vi "main.vi"() -> ()   [LabVIEW 2016]
doc: "Use this template to build a producer/consumer design pattern with events to produce queue items. Use this design pattern instead of the User Interface Event Handler pattern for user interfaces when you want to execute code asynchronously in response to an event without slowing the user interface responsiveness."
uses:
  Microscope_Settings.ctl
  Laser.ctl
  Time_microseconds.ctl
  Phase_Shift.ctl
  Mirror_Voltage.ctl
  Z_Offset.ctl
  Gain.ctl
  Tuneable_Lens_Numeric_Control.ctl
  Piezo_micrometres.ctl
  waveforms.ctl
  Piezo_micrometres_slider_control.ctl
  Mirror_Gain_Slider_Control.ctl
  Tunable_Lens_Slider_Control.ctl
  Desktop/SPIM Controller/functions/Arduino/Old/ArduinoIII Older/MasterArduinoctl.ctl
  Desktop/SPIM Controller/functions/Arduino/Old/ArduinoIII Older/ArduinoII.ctl
panel:
  in  "Experiment Runs":dbl=1.0
  out "error out":errorcluster
  in  "Experiment?":bool
  in  "t2":dbl
  in  "t1":dbl
  in  "COM port":i32
  in  "Mode":T1(ring)
  in  "Number of Repetitions":u16=1 min=1 step=1
  in  "Time Interval  Between Repeats (µS)":T2 step=2
  in  "StopMultiDScan":bool
  in  "StartMultiDScan":bool
  in  "Number of Z Slices":i16=1 min=1 step=1
  in  "Z Mirror Control":enum16{"manual", "automatic"}(ring)
  in  "Apply ex/det correction":enum16{"no", "yes"}(ring)
  out "Z Mirror Voltage":T3 min=-10.0 max=10.0
  out "Adjusted Scan Mirror Voltage":T3 min=-10.0 max=10.0
  in  "set@minZ":bool
  in  "set@maxZ":bool
  in  "@ min Z":T3 min=-10.0 max=10.0
  in  "@ max Z":T3 min=-10.0 max=10.0
  in  "PiezoEndMicrometres":T4 caption="End (µm)" min=0.0 max=100.0
  in  "PiezoStartMicrometres":T4 caption="Start (µm)" min=0.0 max=100.0
  in  "setPiezoEnd":bool
  in  "setPiezoStart":bool
  in  "Lens 2":T5 min=0.0 max=3.0 step=0.0001 scale=0.0..3.0
  in  "Lens 1":T5 min=0.0 max=3.0 step=0.0001 scale=0.0..3.0
  in  "saveMicroscopeSettings":bool
  in  "applyCurrentMicroscopeSettings":bool
  in  "deleteCurrentMicroscopeSettings":bool
  in  "loadMicroscopeSettings":bool
  in  "addMicroscopeSettings":bool
  in  "Z Mirror Gain":T6 min=-10.0 max=10.0 scale=-0.1..0.1
  in  "Mirror Offset":dbl(slide) min=-10.0 max=10.0 step=0.01 scale=0.0..1.8
  in  "Laser":T7
  in  "Piezo Position (µm)":T8 min=0.0 max=100.0 scale=0.0..100.0
  in  "Mirror Voltage":dbl(slide) min=-10.0 max=10.0 step=0.01 scale=-4.0..5.0
  in  "setPosition2":bool
  in  "setPosition1":bool
  in  "Z offset 2":T9
  in  "Z offset 1":T9
  in  "Scan Mirror 2":T3 min=-10.0 max=10.0
  in  "Scan Mirror 1":T3 min=-10.0 max=10.0
  in  "setScanMirrorMin":bool
  in  "setScanMirrorMax":bool
  in  "MinScanMirror":T3 caption="Min" min=-10.0 max=10.0
  in  "MaxScanMirror":T3 caption="Max" min=-10.0 max=10.0
  in  "Offset":T3 min=-10.0 max=10.0
  in  "Amplitude":T3 min=-10.0 max=10.0
  in  "Phase Shift (µS)":i32(slide) scale=-5000.0..1000.0
  in  "Sweep Interval (µS)":T2 step=2
  in  "Sweep Time (µS)":T2 step=20
  in  "Microscope Settings":T10[](array[typedef]) {"Number Z Slices" min=1 step=1; "Piezo End (µm)" min=0.0 max=100.0; "Piezo Start (µm)" min=0.0 max=100.0; "Beam @ max Z" min=-10.0 max=10.0; "Beam @ min Z" min=-10.0 max=10.0; "Tuneable Lens 2" min=0.0 max=3.0 step=0.0001; "Tuneable Lens 1" min=0.0 max=3.0 step=0.0001; "Scan Mirror Position 2" min=-10.0 max=10.0; "Scan Mirror Position 1" min=-10.0 max=10.0; "Scan Mirror Amplitude" min=-10.0 max=10.0; "Scan Mirror Min" min=-10.0 max=10.0; "Scan Mirror Max" min=-10.0 max=10.0; "Sweep Interval (µS)" step=2; "Sweep Time (µS)" step=2}
  in  "Sample Rate (kHz)":i32
  in  "StopSinglePlaneScan":bool
  in  "StartSinglePlaneScan":bool
  in  "exit":bool
  # "Piezo Settings"
  # "Scan Mirror Settings"
  # "Z Mirror Local Settings"
  # "Single Plane Scan"
  # "Multidimensional Scan"
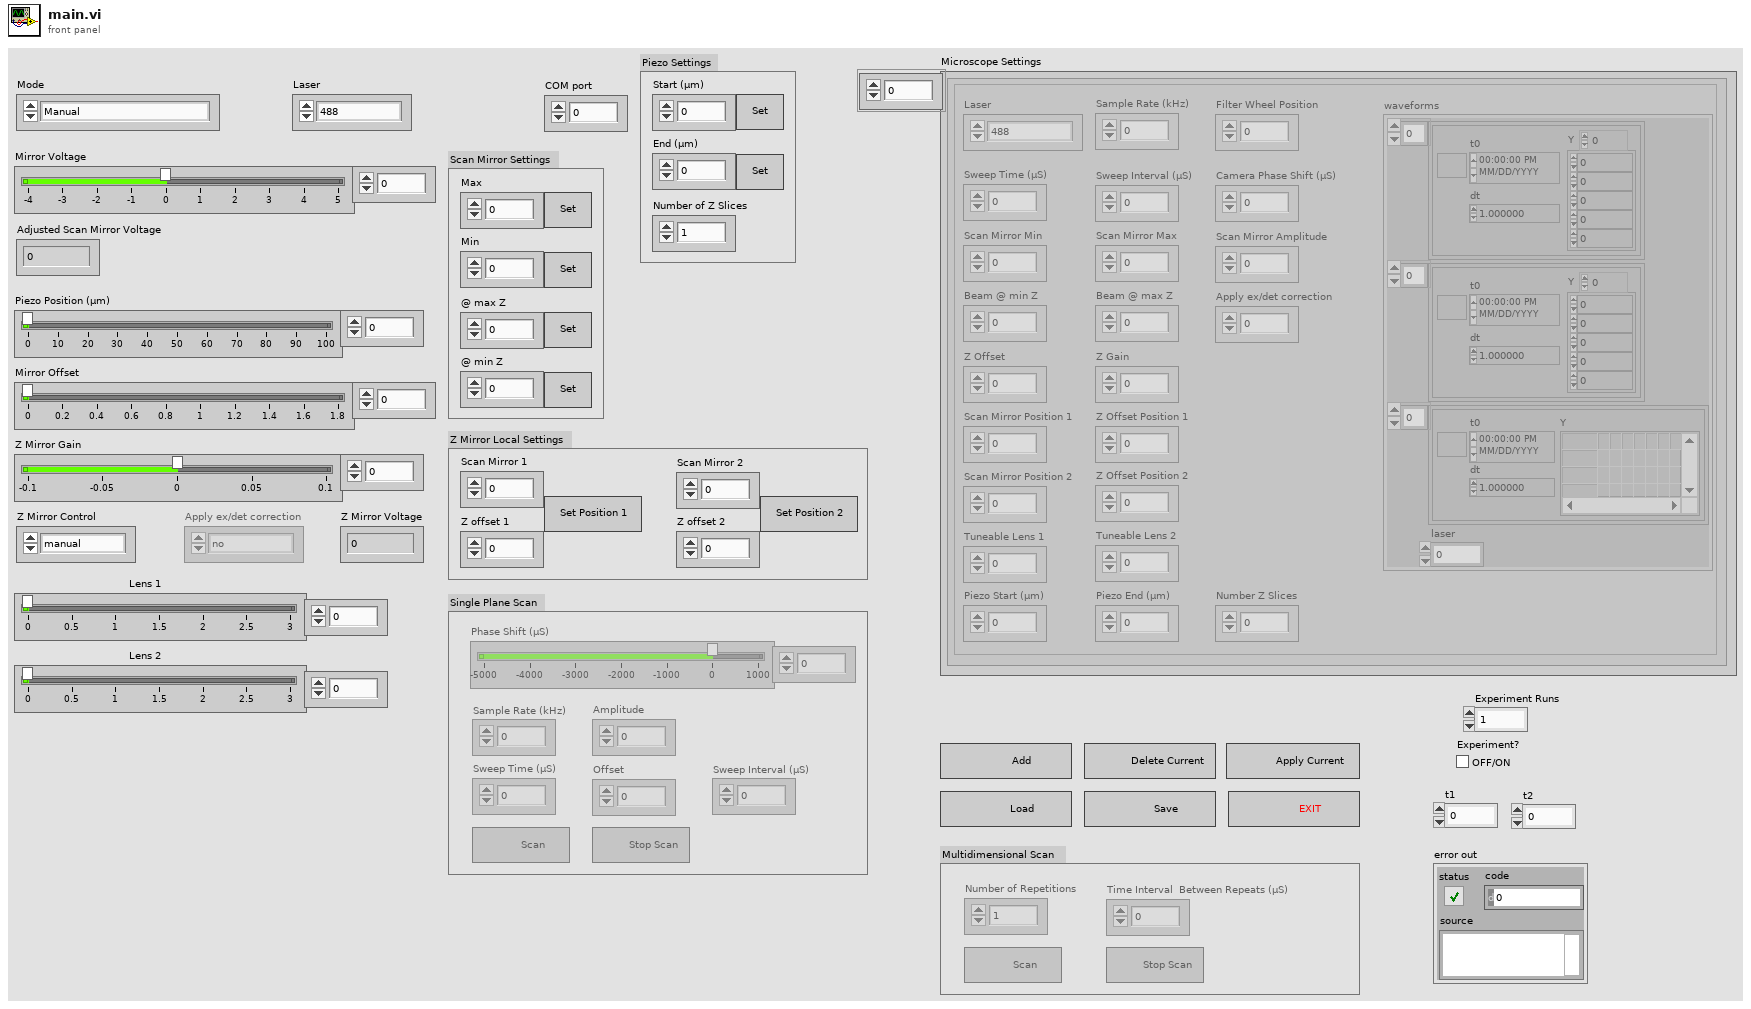
[diagram p1: front panel]
types:
  T1 = enum8{"Manual", "Single Plane Scan", "Multi-Dimensional Scan"}
  T2 = typedef "Time_microseconds.ctl" = u32
  T3 = typedef "Mirror_Voltage.ctl" = dbl
  T4 = typedef "Piezo_micrometres.ctl" = dbl
  T5 = typedef "Tunable_Lens_Slider_Control.ctl" = dbl
  T6 = typedef "Mirror_Gain_Slider_Control.ctl" = dbl
  T7 = typedef "Laser.ctl" = enum16{"488", "561"}
  T8 = typedef "Piezo_micrometres_slider_control.ctl" = dbl
  T9 = typedef "Z_Offset.ctl" = dbl
  T10 = typedef "Microscope_Settings.ctl" = cluster{"Laser":T7, "Sweep Time (µS)":T2, "Sweep Interval (µS)":T2, "Sample Rate (kHz)":dbl, "Camera Phase Shift (µS)":T11, "Scan Mirror Max":T3, "Scan Mirror Min":T3, "Scan Mirror Amplitude":T3, "Z Offset":T9, "Z Gain":T12, "Scan Mirror Position 1":T3, "Z Offset Position 1":T9, "Scan Mirror Position 2":T3, "Z Offset Position 2":T9, "Tuneable Lens 1":T13, "Tuneable Lens 2":T13, "Beam @ min Z":T3, "Beam @ max Z":T3, "Piezo Start (µm)":T4, "Piezo End (µm)":T4, "Number Z Slices":i16, "Filter Wheel Position":i32, "Apply ex/det correction":u16, "waveforms":T14}
  T11 = typedef "Phase_Shift.ctl" = i32
  T12 = typedef "Gain.ctl" = dbl
  T13 = typedef "Tuneable_Lens_Numeric_Control.ctl" = dbl
  T14 = typedef "waveforms.ctl" = cluster{waveform(dbl)[], waveform(dbl)[], digitalwaveform[], "laser":i32}
  T15 = typedef "ArduinoII.ctl" = enum16{"Timed XP", "Z_UP", "Z_DOWN", "XY_UP", "XY_LEFT", "XY_RIGHT", "XY_DOWN", "Stop", "Idle", "power_reset", "power_is_set_on", "power_is_set_off", "curr_1_changed", "curr_2_changed", "curr_3_changed", "curr_4_changed"}
  T16 = typedef "MasterArduinoctl.ctl" = cluster{"Current":cluster{"curr_1_value":dbl, "curr_2_value":dbl, "curr_3_value":dbl, "curr_4_value":dbl, "Write All":bool}, "Boolean Set":cluster{"XY Up":bool, "XY Down":bool, "XY Left":bool, "XY Right":bool, "Z Up":bool, "Z Down":bool}, "Cluster":cluster{"XY Up":dbl, "XY Down":dbl, "XY Left":dbl, "XY Right":dbl, "Z Up":dbl, "Z Down":dbl}, "Timing":cluster{"t1":dbl, "t2":dbl, "Timed Experiment":bool}, "Power":cluster{"Power ON":bool, "Power OFF":bool}}
  T17 = enum8{"Enabled", "Disabled", "Disabled and Grayed Out"}
  T18 = enum16{"deny read/write", "deny write-only", "deny none"}
  T19 = enum16{"open", "replace", "create", "open or create", "replace or create", "replace or create with confirmation"}
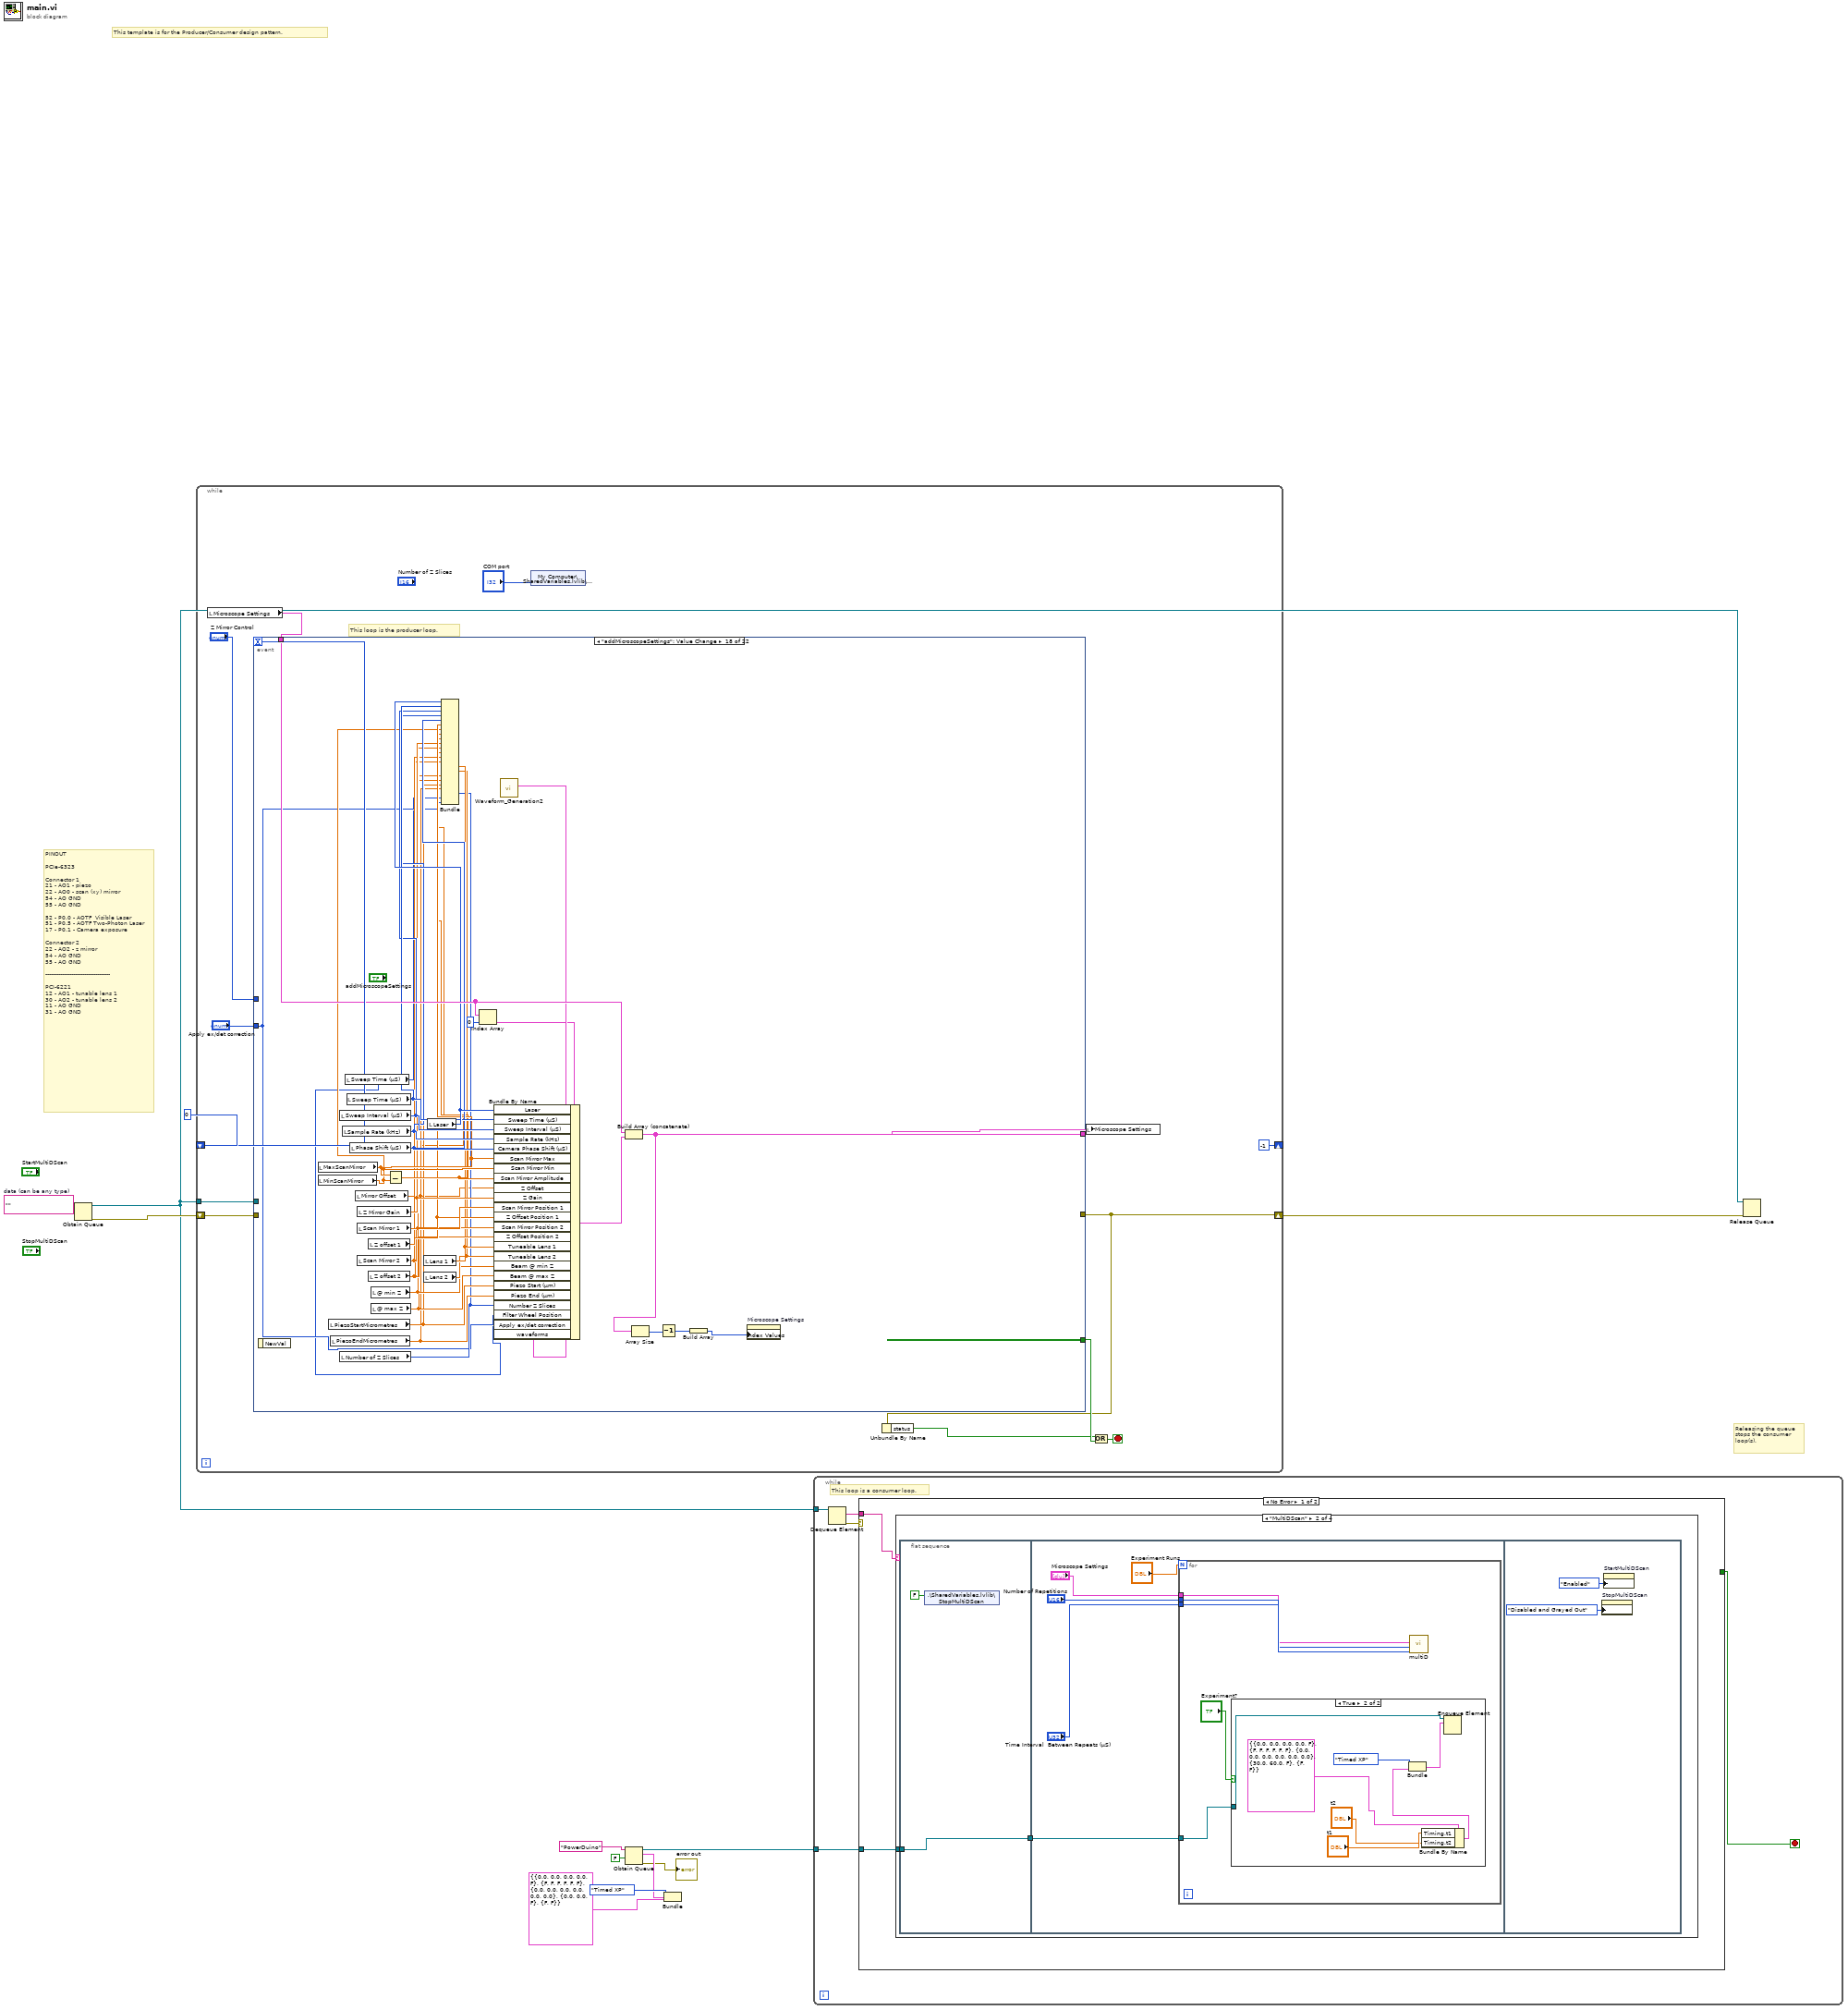
[diagram p0: block diagram]
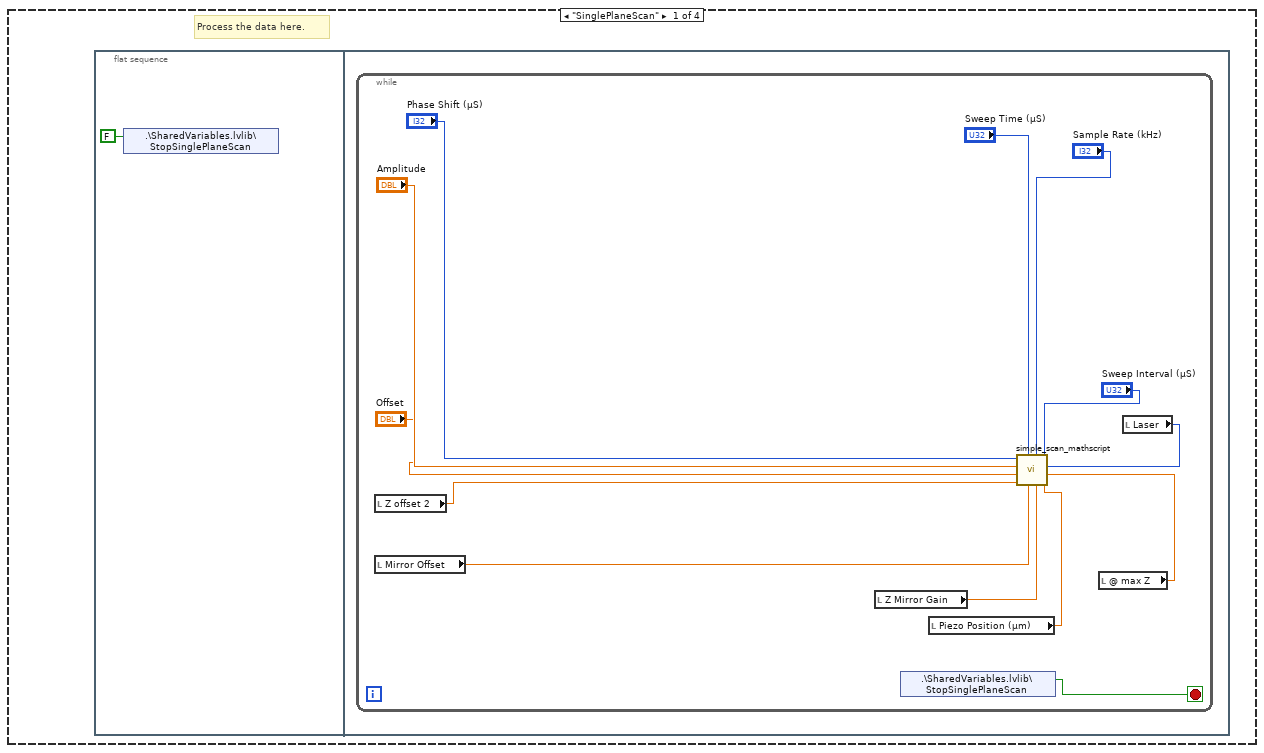
[diagram p2: hidden frame]
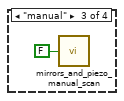
[diagram p4: hidden frame]
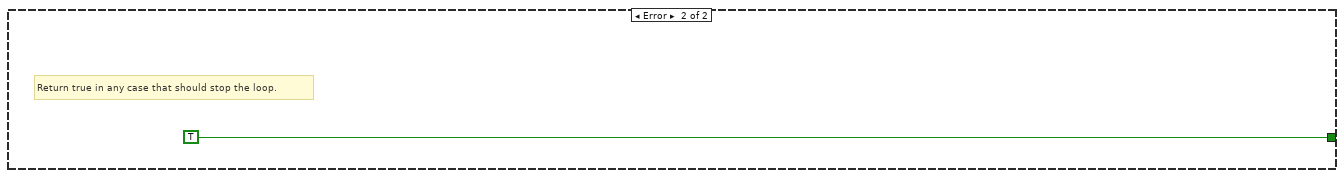
[diagram p6: hidden frame]
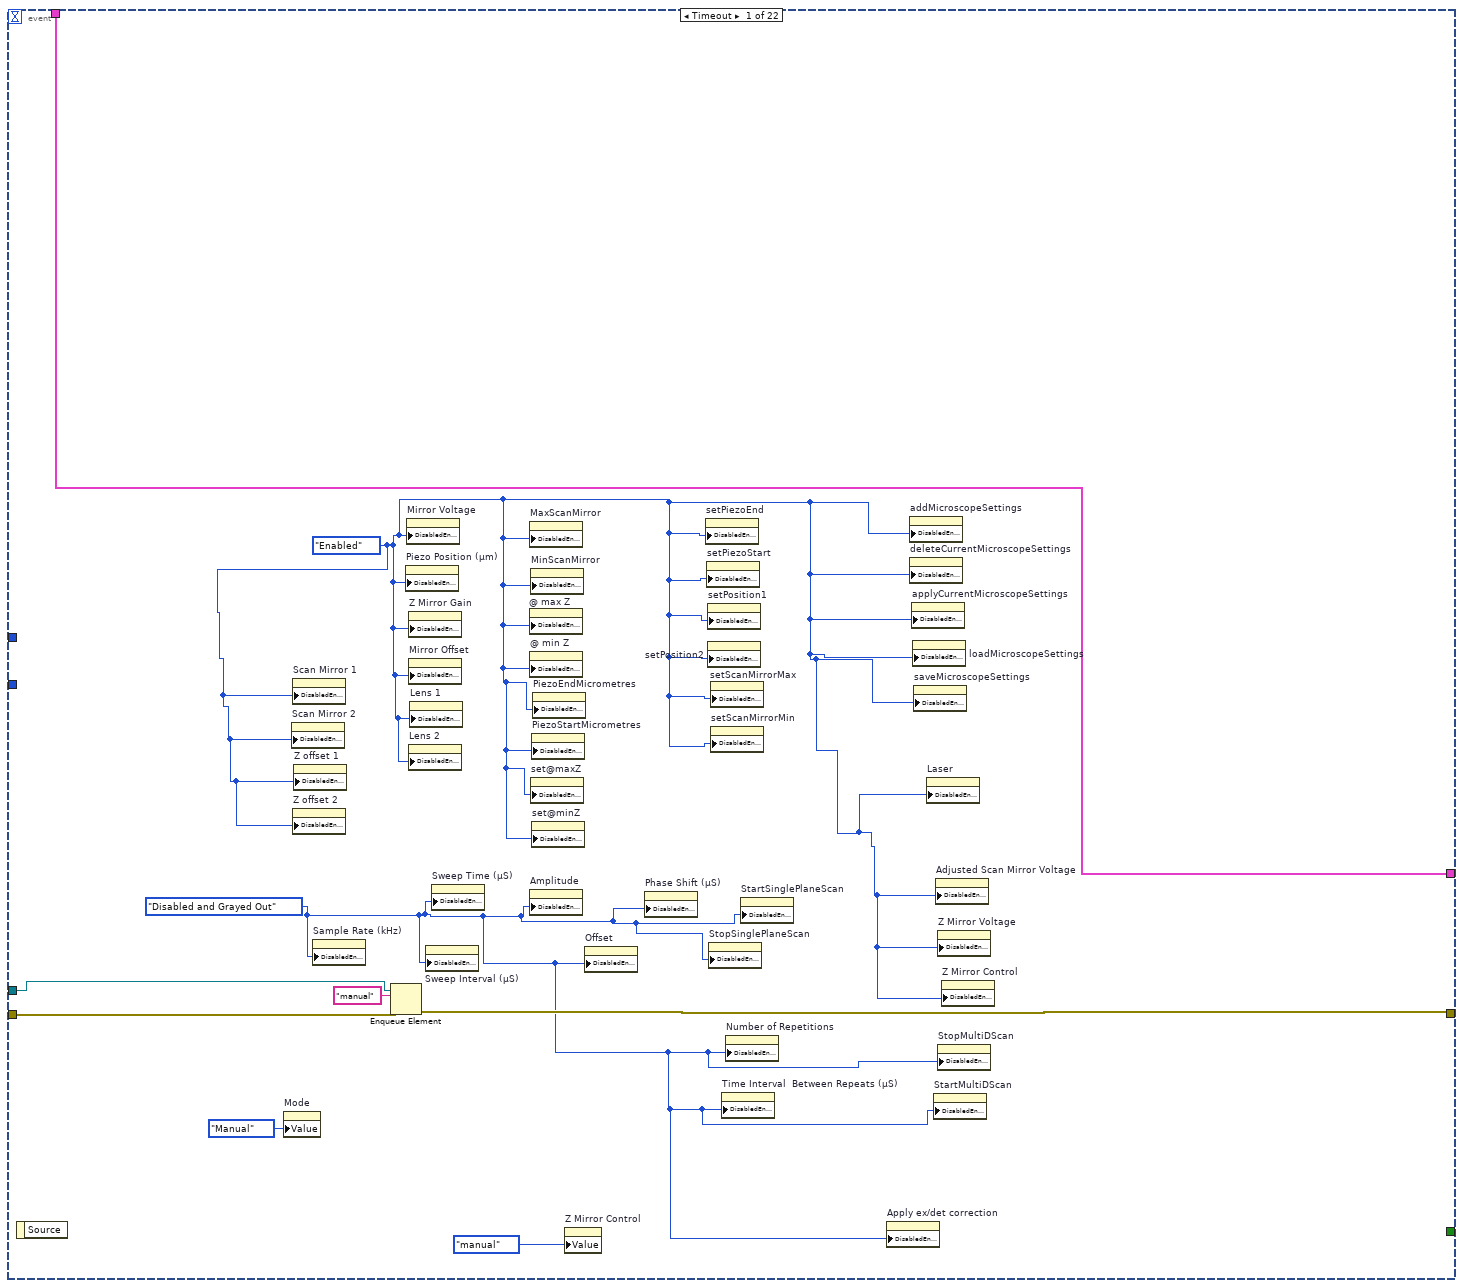
[diagram p7: hidden frame]
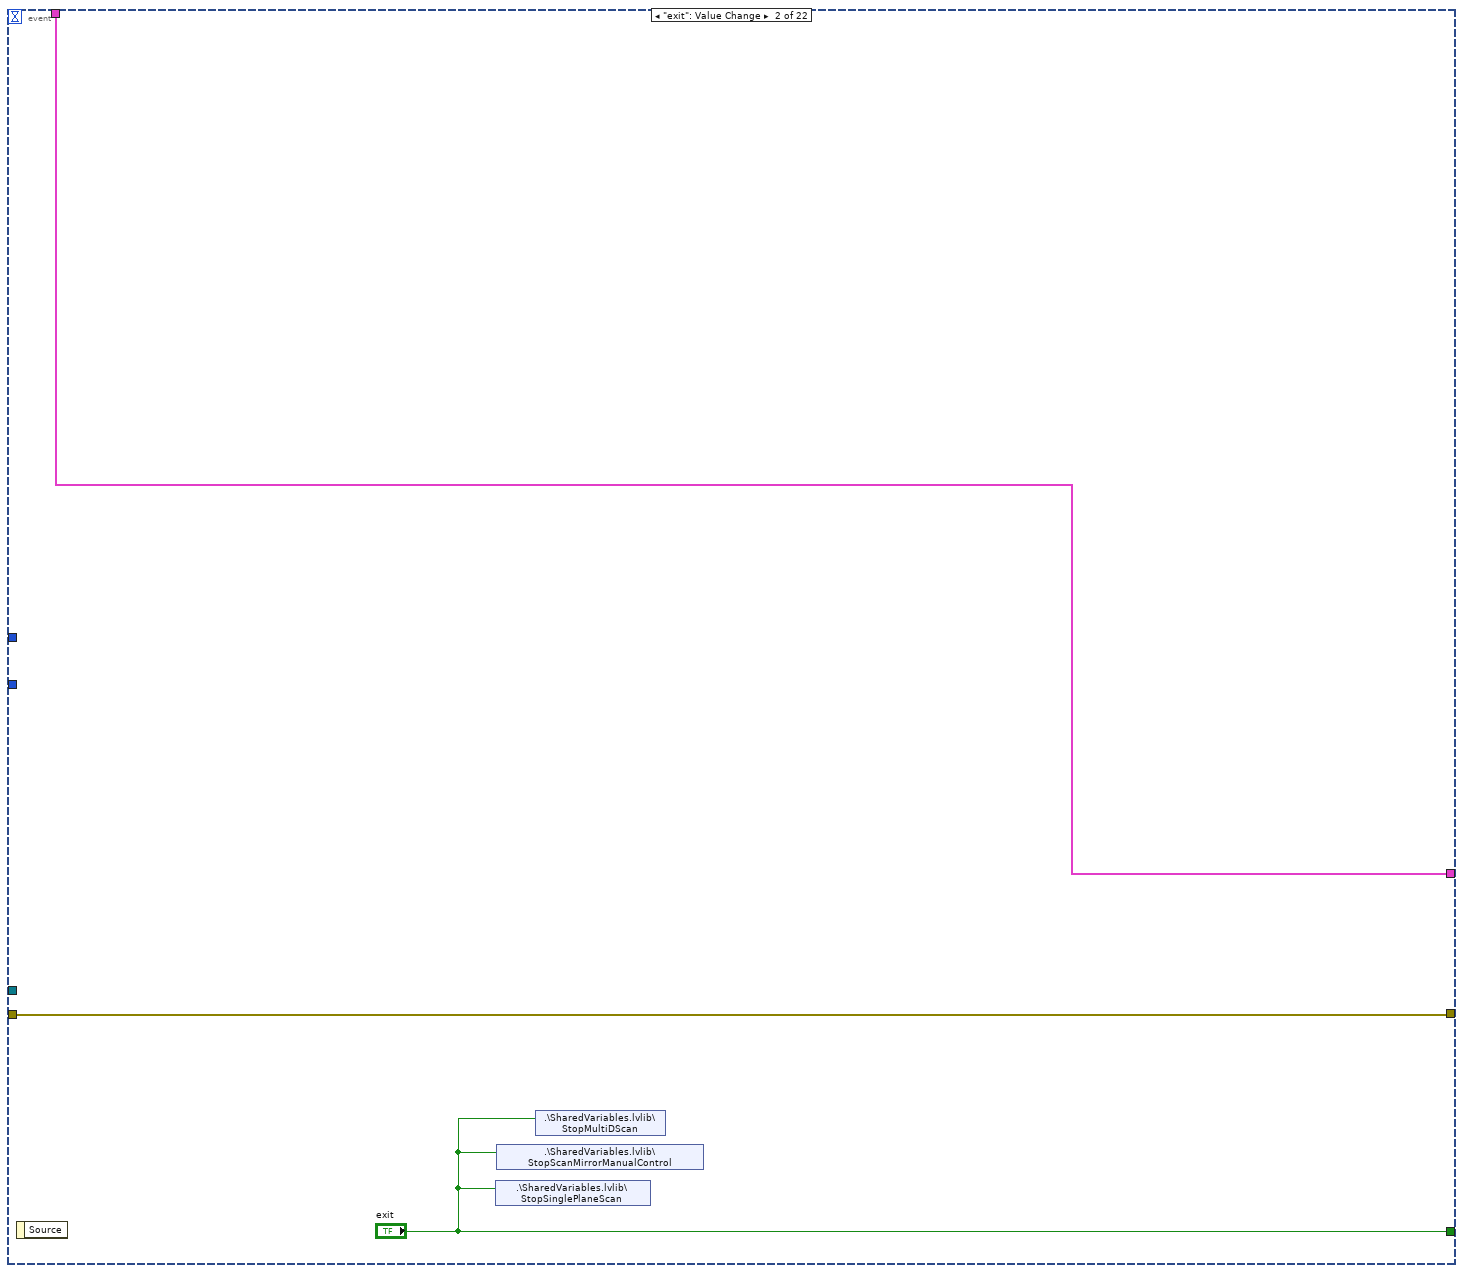
[diagram p8: hidden frame]
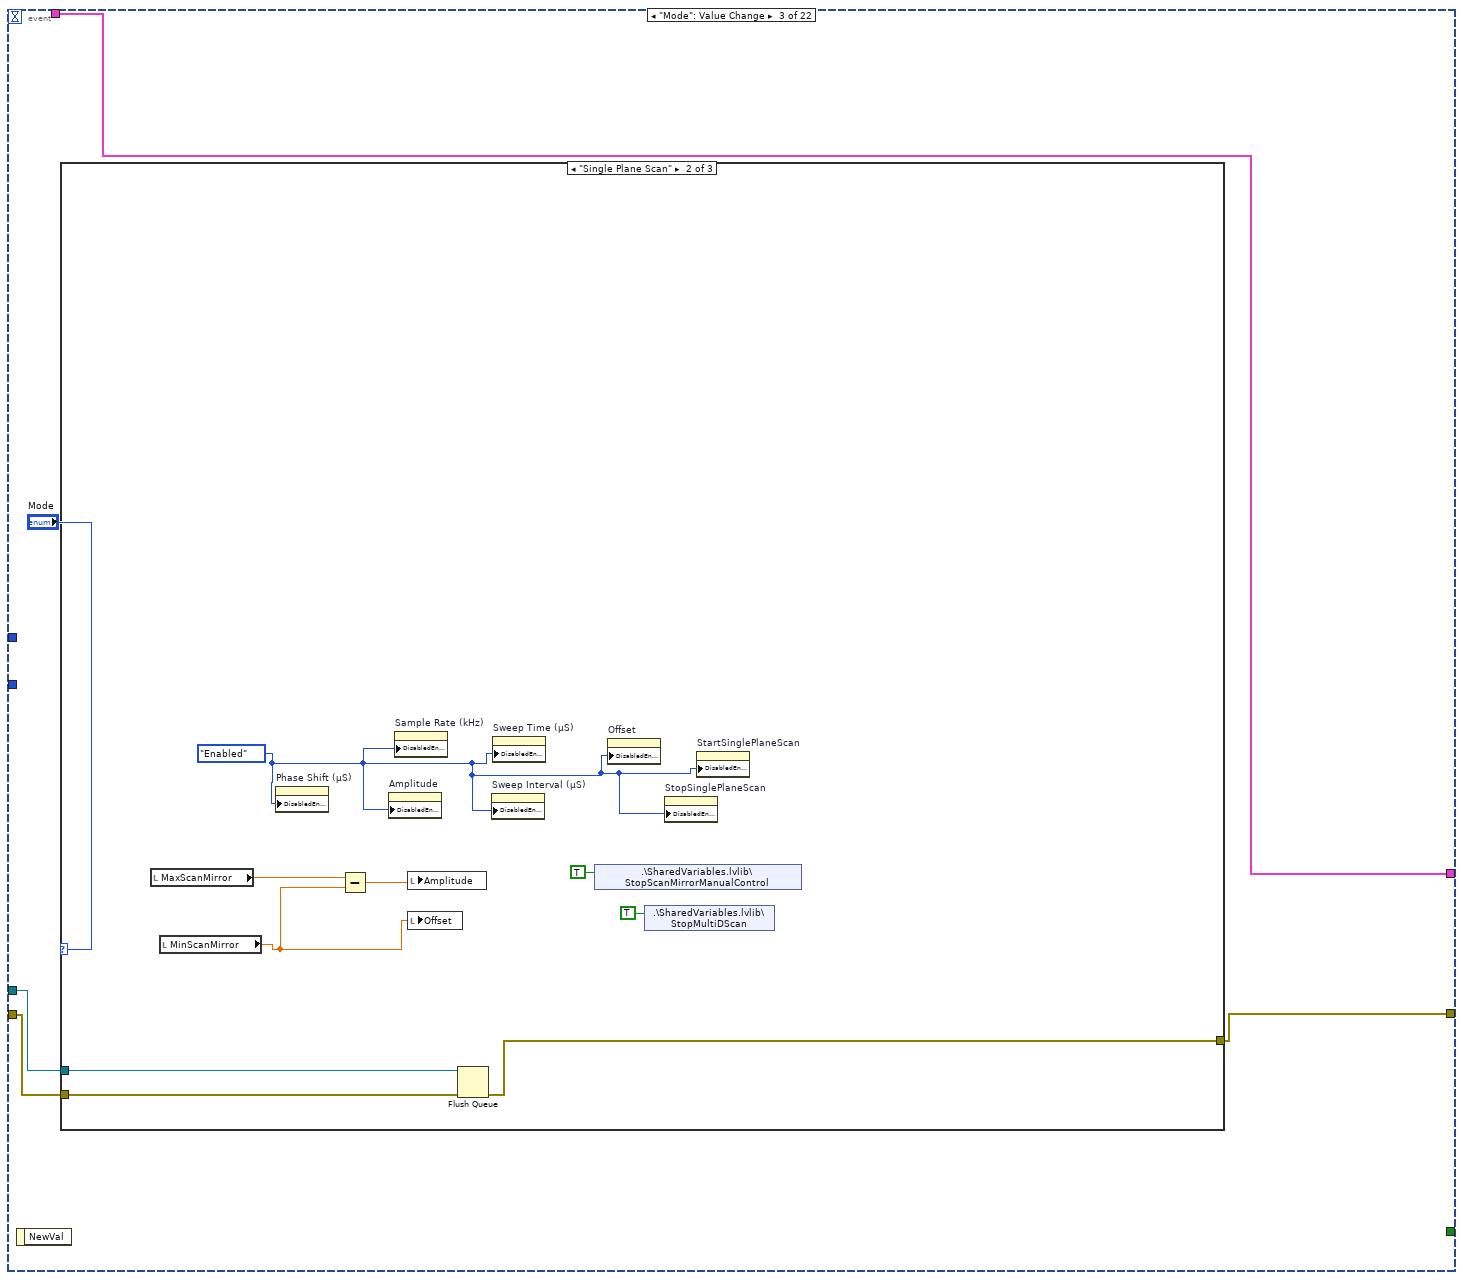
[diagram p9: hidden frame]
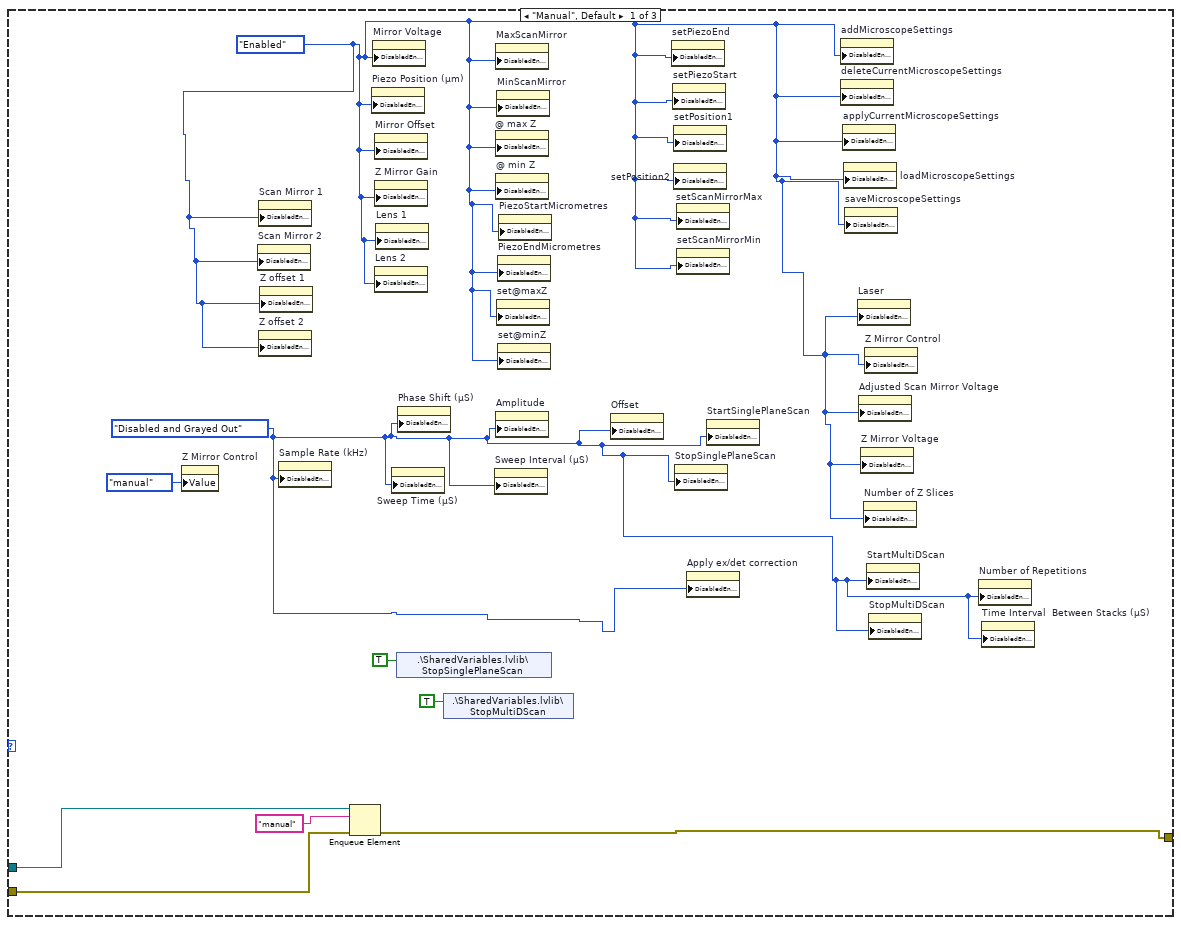
[diagram p10: hidden frame]
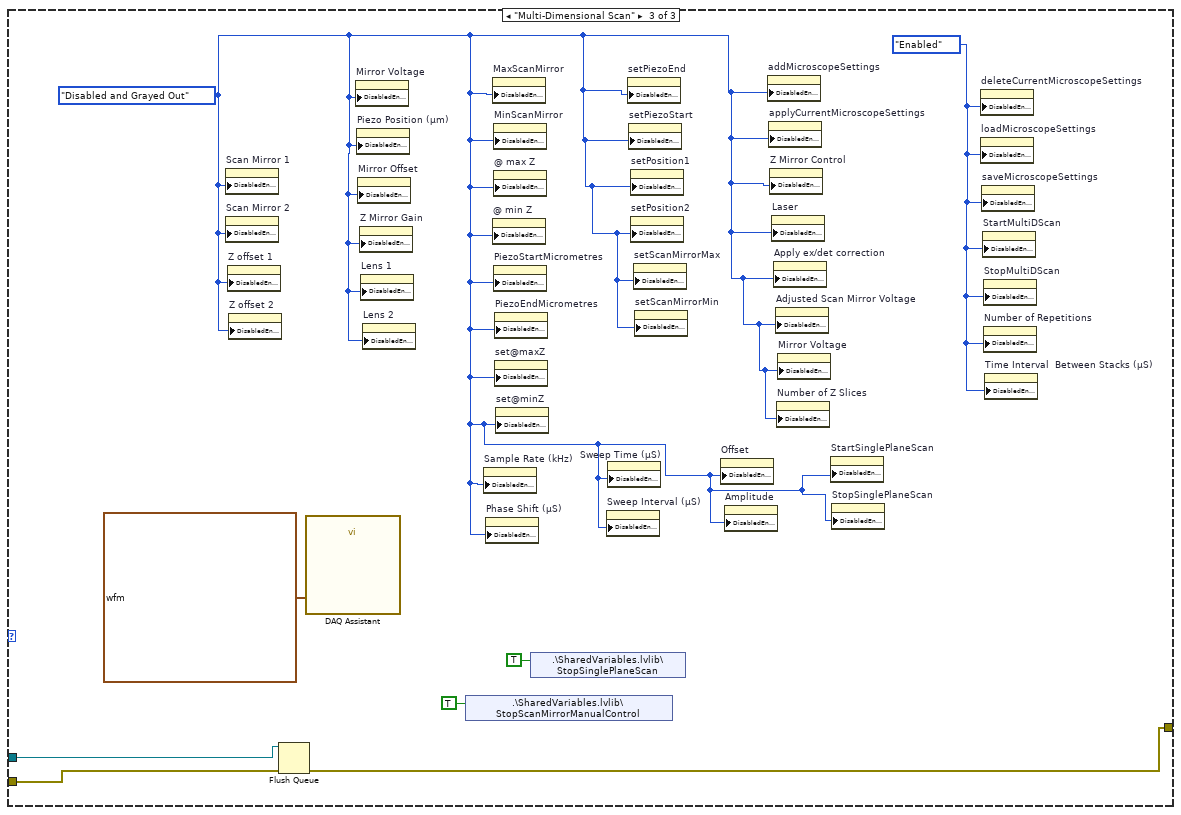
[diagram p11: hidden frame]
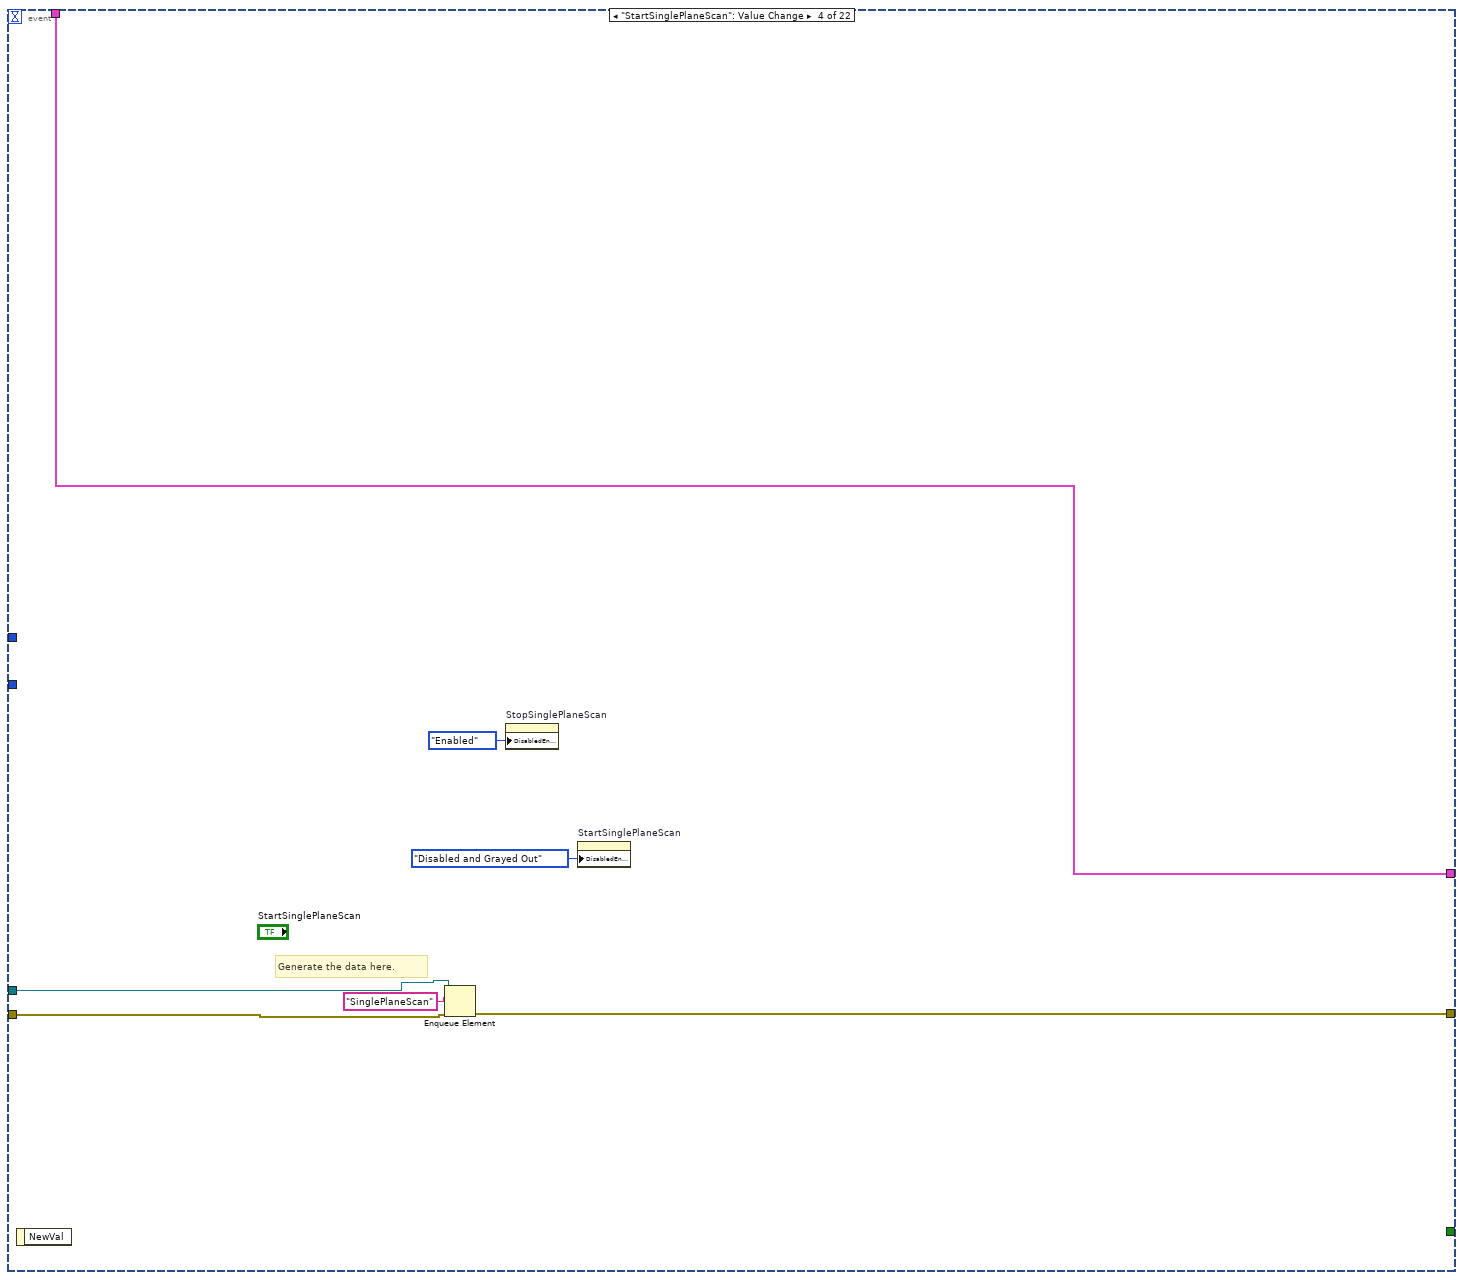
[diagram p12: hidden frame]
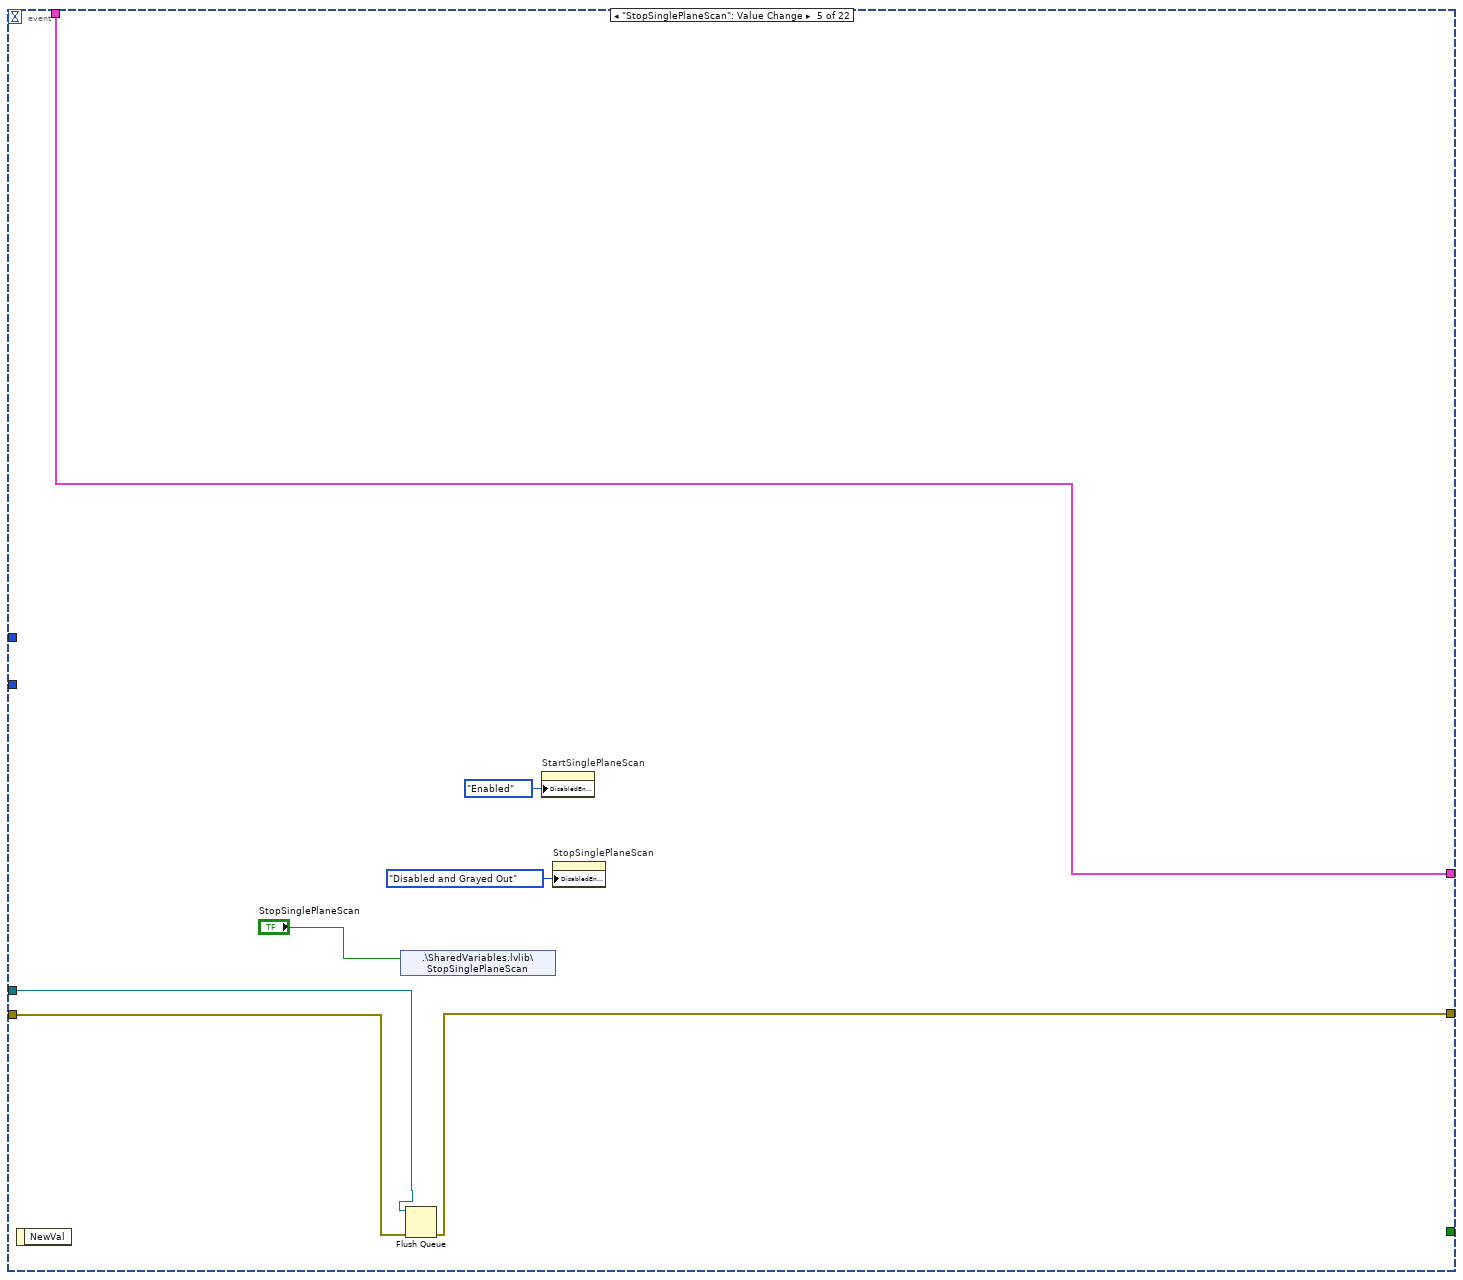
[diagram p13: hidden frame]
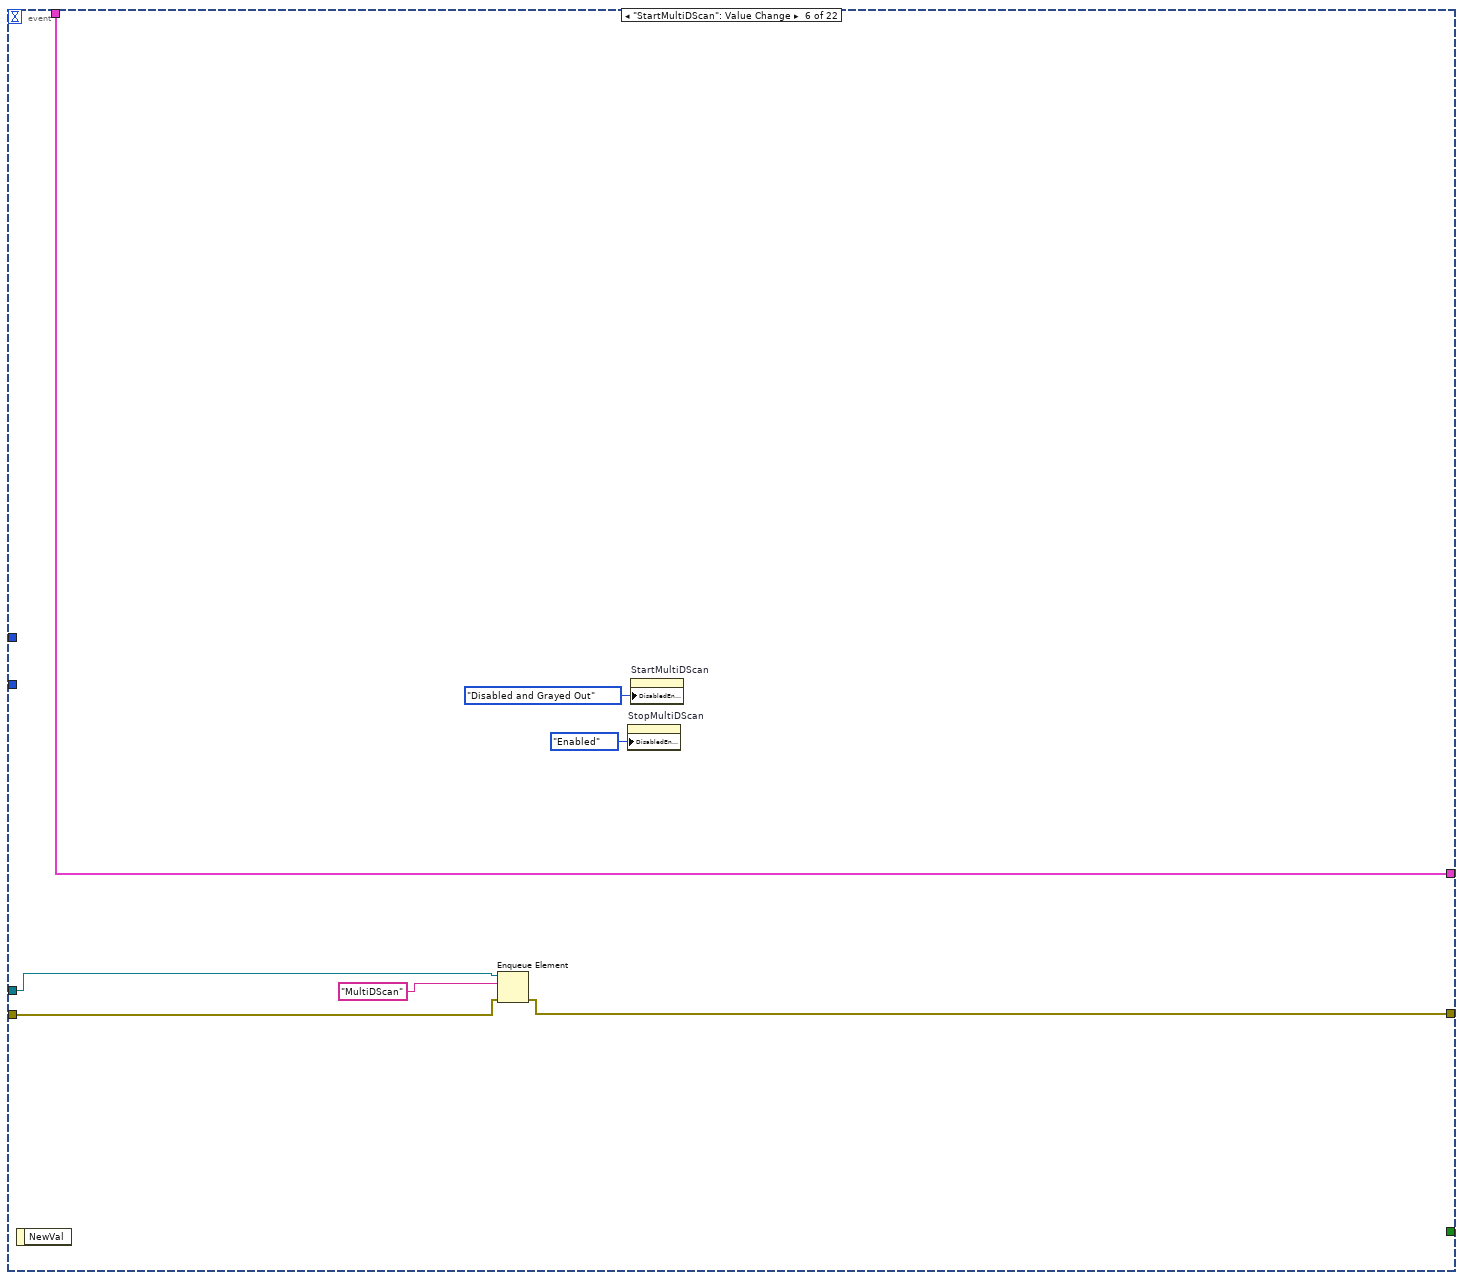
[diagram p14: hidden frame]
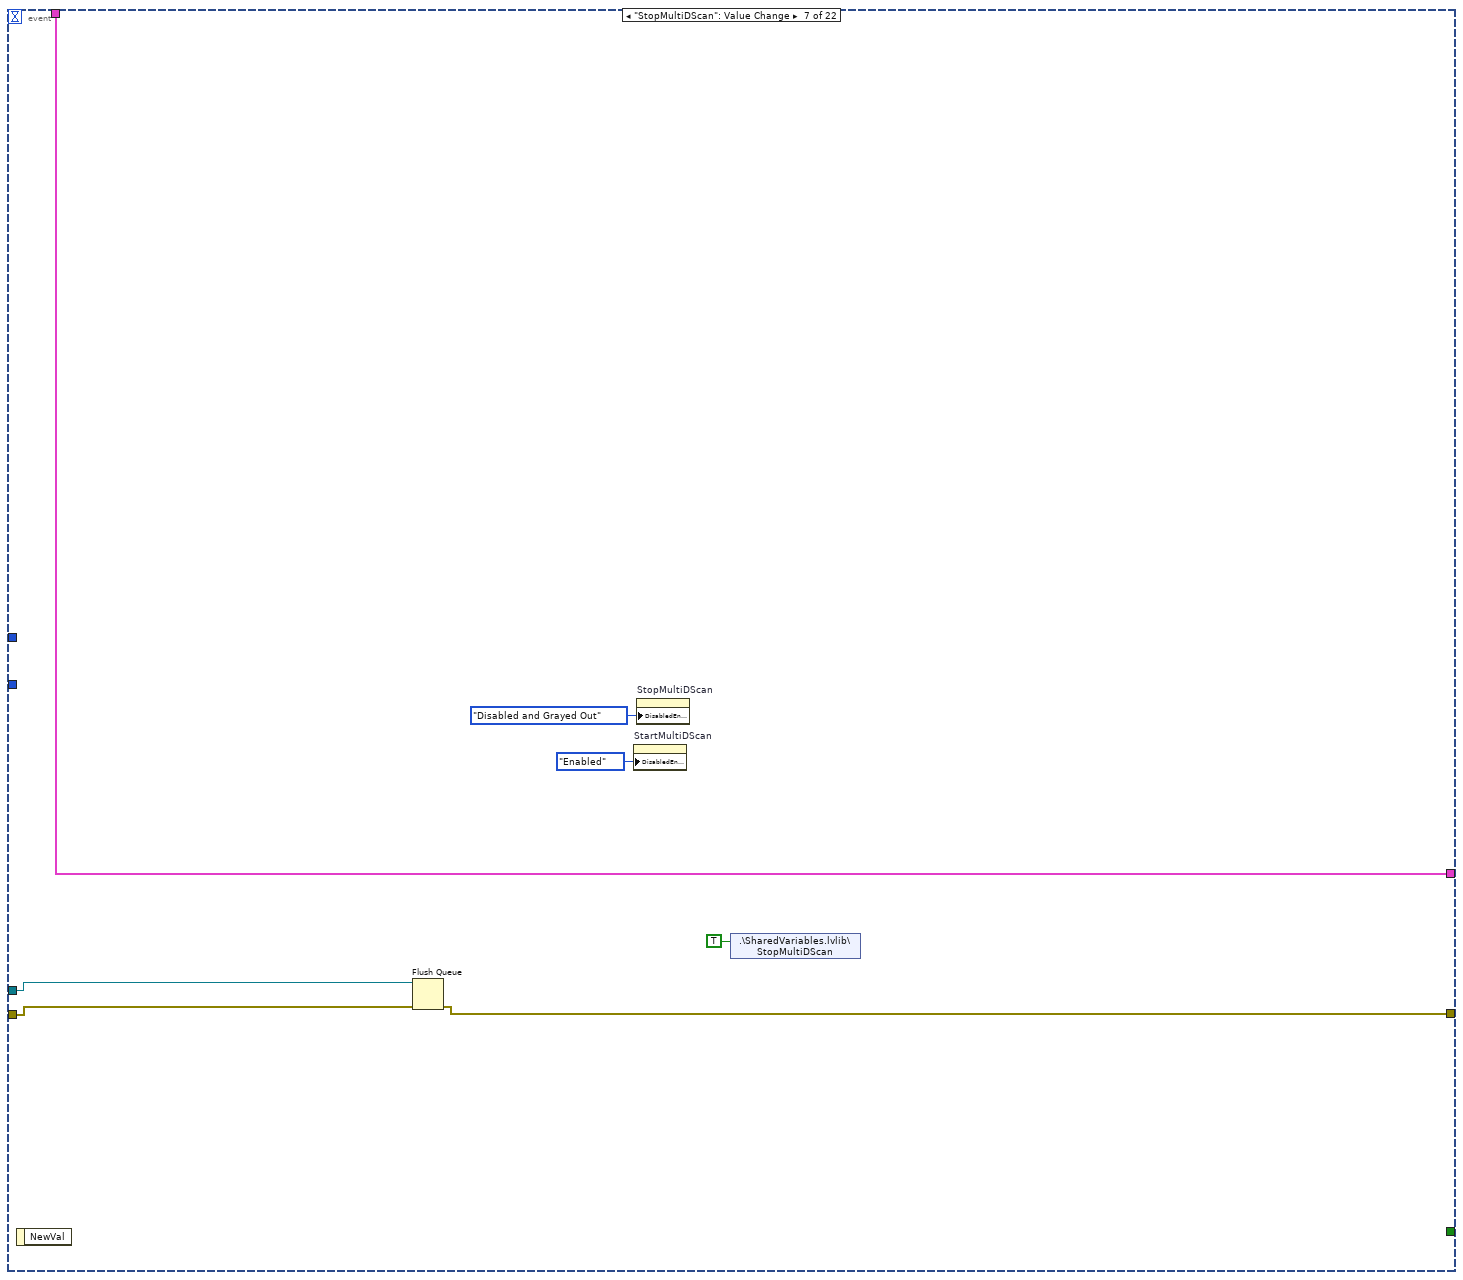
[diagram p15: hidden frame]
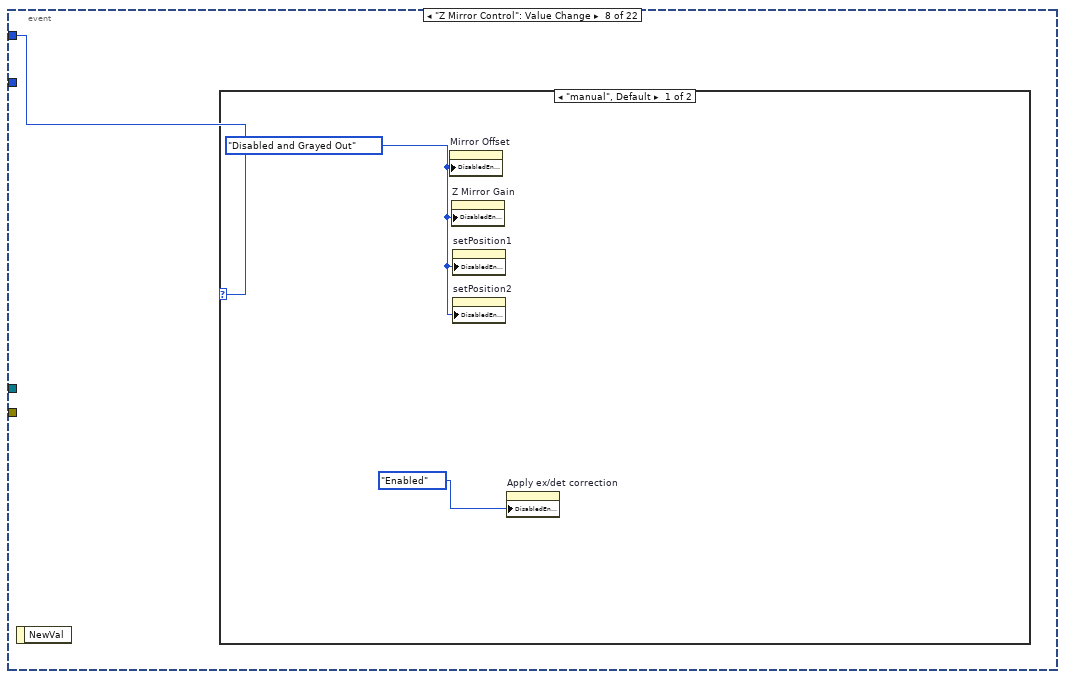
[diagram p16: hidden frame]
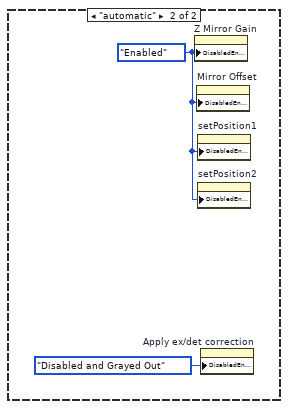
[diagram p17: hidden frame]
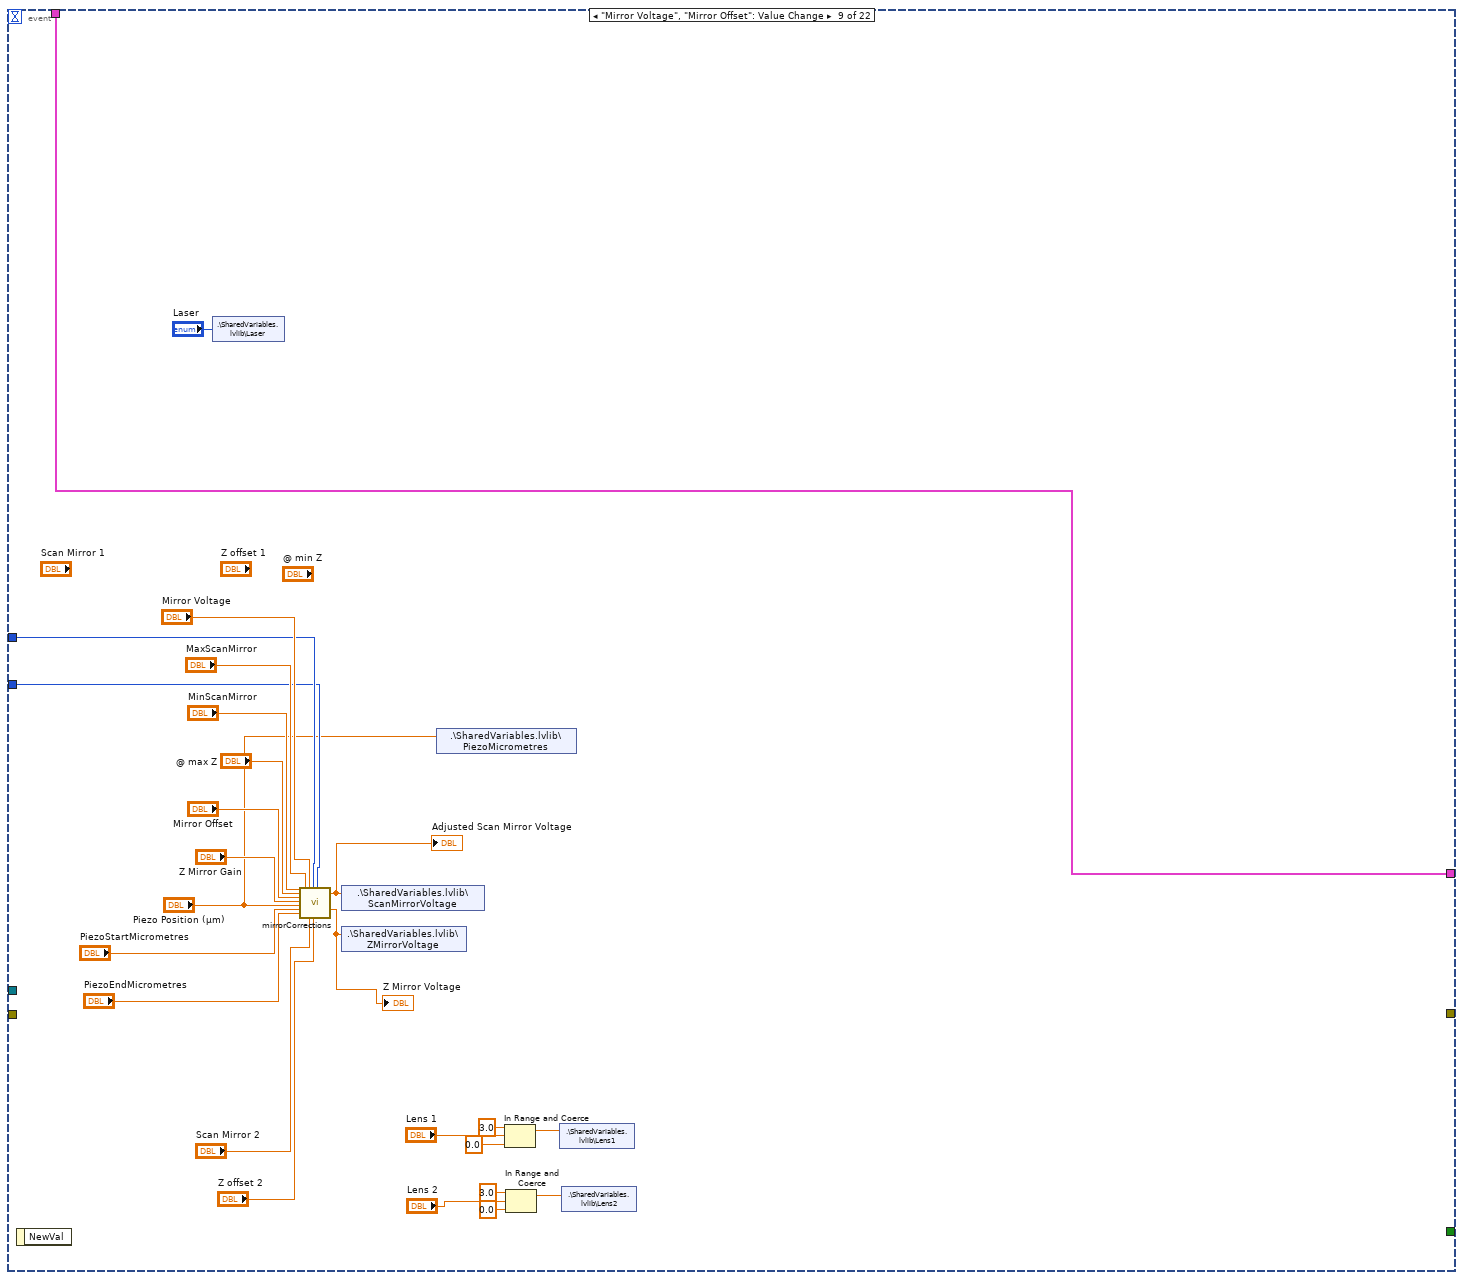
[diagram p18: hidden frame]
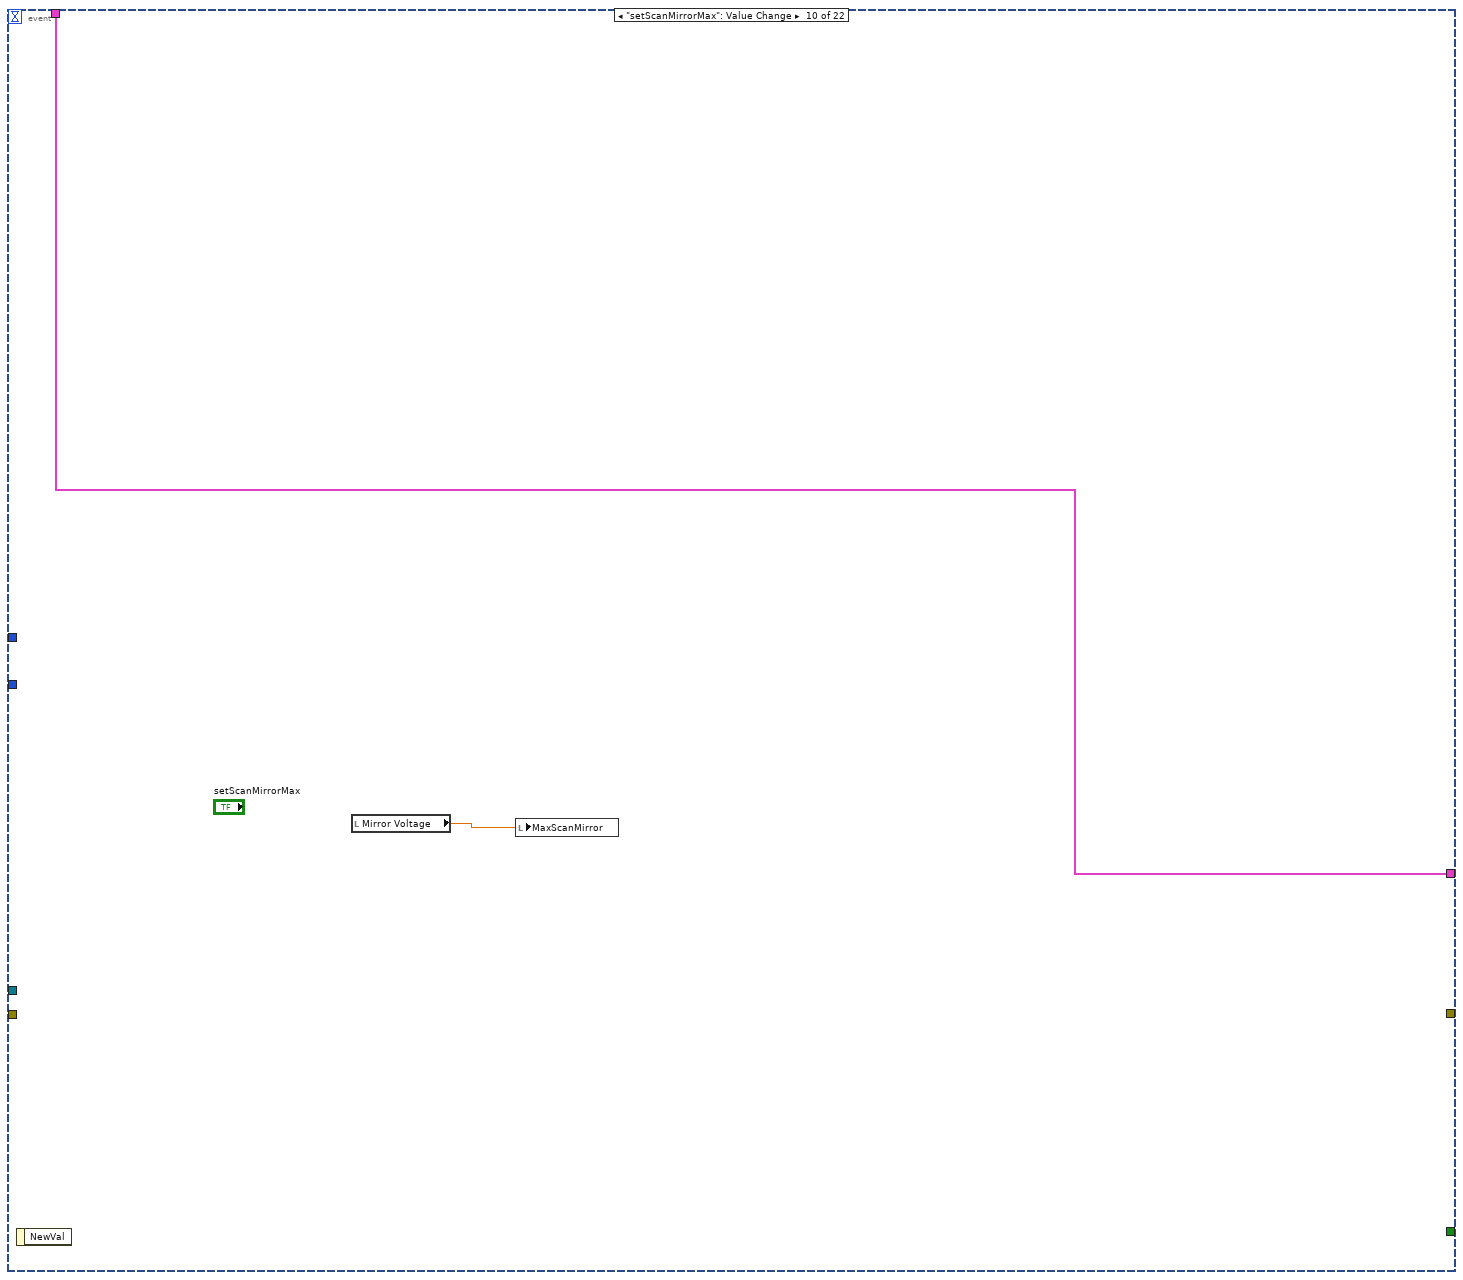
[diagram p19: hidden frame]
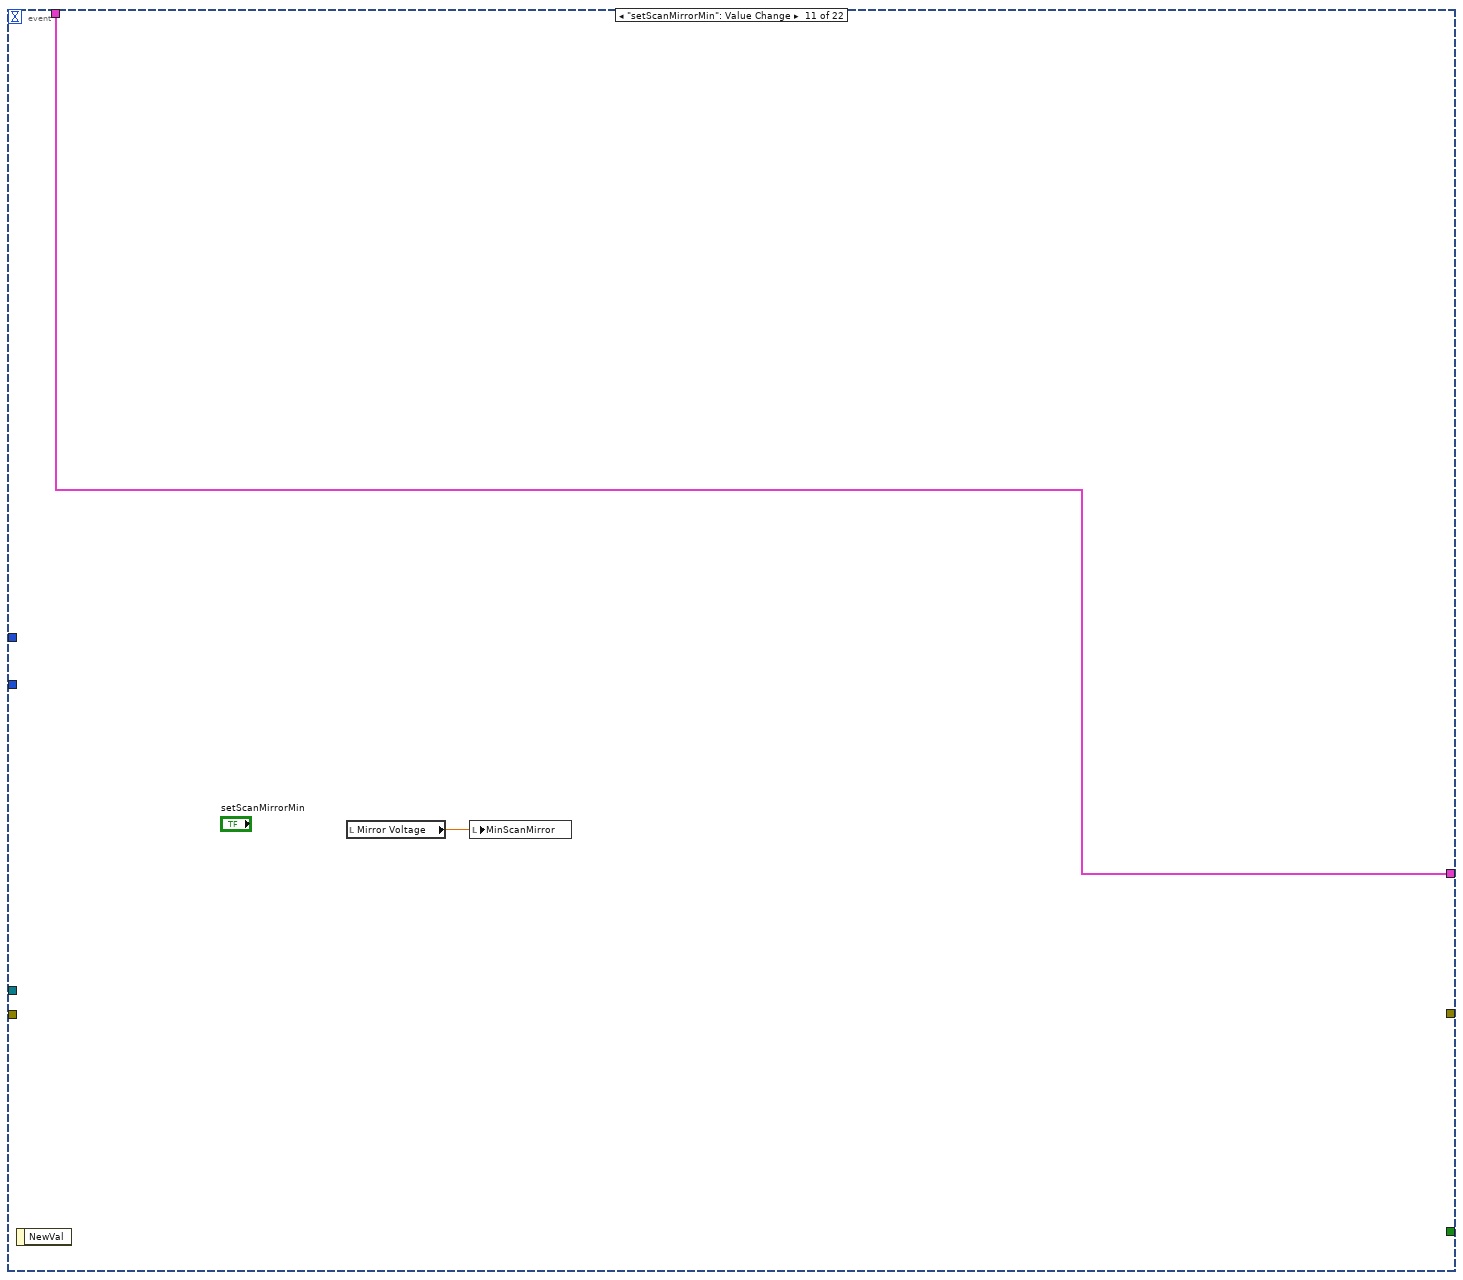
[diagram p20: hidden frame]
diagram:
  w10 = ""  # data (can be any type)
  # "PINOUT\n\nPCIe-6323\n\nConnector 1\n21 - AO1 - piezo\n22 - AO0 - scan (xy) mirror\n54 - AO GND\n55 - AO GND\n\n52 - P0.0 - AOTF  Visible Laser\n51 - P0.5 - AOTF Two-Photon Laser\n17 - P0.1 - Camera exposure\n\nConnector 2\n22 - AO2 - z mirror\n54 - AO GND\n55 - AO GND\n\n-----------------------------------\n\nPCI-6221\n12 - AO1 - tunable lens 1\n30 - AO2 - tunable lens 2\n11 - AO GND\n31 - AO GND"
  # "Releasing the queue stops the consumer loop(s)."
  # "This template is for the Producer/Consumer design pattern."
  n1 = Obtain Queue(element data type=w10) -> (queue out=w8:refnum<queue>, error out=w12:errorcluster)  [unwired: 4 in, 1 out]
  n2 = while {
    shift-right: [w21] -> w11
    shift-left: w12 -> [w24]
    tunnel: w8 -> [w25]
    shift-right: [-1] -> _
    shift-left: 0 -> [w19]
    stop <- w22 stop-if-true
    # "This loop is the producer loop."
    n3 = local read "Microscope Settings"() -> (w17:T10[])
    n4 = event shown="[17] \"addMicroscopeSettings\": Value Change" {
      selector: _ -> [_ _ _ _ _ _ _ _ _ _ _ _ _ _ _ _ _ _ _ _ _ _]
      dyn-events: _ -> [_ _ _ _ _ _ _ _ _ _ _ _ _ _ _ _ _ _ _ _ _ _]
      timeout: w19 -> [_ _ _ _ _ _ _ _ _ _ _ _ _ _ _ _ _ _ _ _ _ _]
      tunnel: w25 -> [w34 _ w41 w75 w81 w89 w96 _ _ _ _ _ _ _ _ _ _ _ _ _ _ _]
      tunnel: w24 -> [w33 w37 w40 w74 w80 w88 w95 _ _ _ _ _ _ _ _ _ _ _ _ _ _ _]
      tunnel: [w32 w37 w39 w73 w79 w87 w94 _ _ _ _ _ _ _ _ _ _ _ _ _ _ _] -> w21
      tunnel: [_ "exit" _ _ _ _ _ _ _ _ _ _ _ _ _ _ _ _ _ _ _ _] -> w23
      tunnel: [w30 w36 w38 w71 w78 w86 w93 _ w126 w127 w129 w131 w134 w137 w139 w141 w143 w172 w178 w213 w218 w241] -> w14
      tunnel: w17 -> [w30 w36 w38 w71 w78 w86 w93 _ w126 w127 w129 w131 w134 w137 w139 w141 w143 w171 w177 w213 w219 w241]
      tunnel: "Z Mirror Control" -> [_ _ _ _ _ _ _ w97 w115 _ _ _ _ _ _ _ _ _ _ _ _ _]
      tunnel: "Apply ex/det correction" -> [_ _ _ _ _ _ _ _ w114 _ _ _ _ _ _ _ _ w150 _ _ _ _]
      event Timeout {
        w29 = T17."Enabled" ("Disabled")
        w27 = T17."Disabled and Grayed Out" ("Disabled")
        n5 = event-data() -> ()  [unwired: 1 in, 1 out]
        n6 = property on="Mode" class="Enum (strict)"("Value"=T1."Manual" ("Mode")) -> ()  [unwired: 2 in, 2 out]
        n7 = property on="Scan Mirror 2" class="DigNum (strict)"("DisabledEnum"=w29) -> ()  [unwired: 2 in, 2 out]
        n8 = property on="Scan Mirror 1" class="DigNum (strict)"("DisabledEnum"=w29) -> ()  [unwired: 2 in, 2 out]
        n9 = property on="Z offset 2" class="DigNum (strict)"("DisabledEnum"=w29) -> ()  [unwired: 2 in, 2 out]
        n10 = property on="Z offset 1" class="DigNum (strict)"("DisabledEnum"=w29) -> ()  [unwired: 2 in, 2 out]
        n11 = property on="Sample Rate (kHz)" class="DigNum (strict)"("DisabledEnum"=w27) -> ()  [unwired: 2 in, 2 out]
        n12 = Enqueue Element(queue=w34, element="manual", error in (no error)=w33) -> (error out=w32:errorcluster)  [unwired: 1 in, 2 out]
        n13 = property on="Piezo Position (µm)" class="Slide (strict)"("DisabledEnum"=w29) -> ()  [unwired: 2 in, 2 out]
        n14 = property on="Mirror Voltage" class="Slide (strict)"("DisabledEnum"=w29) -> ()  [unwired: 2 in, 2 out]
        n15 = property on="Z Mirror Gain" class="Slide (strict)"("DisabledEnum"=w29) -> ()  [unwired: 2 in, 2 out]
        n16 = property on="Mirror Offset" class="Slide (strict)"("DisabledEnum"=w29) -> ()  [unwired: 2 in, 2 out]
        n17 = property on="Lens 2" class="Slide (strict)"("DisabledEnum"=w29) -> ()  [unwired: 2 in, 2 out]
        n18 = property on="Lens 1" class="Slide (strict)"("DisabledEnum"=w29) -> ()  [unwired: 2 in, 2 out]
        n19 = property on="Sweep Interval (µS)" class="DigNum (strict)"("DisabledEnum"=w27) -> ()  [unwired: 2 in, 2 out]
        n20 = property on="Sweep Time (µS)" class="DigNum (strict)"("DisabledEnum"=w27) -> ()  [unwired: 2 in, 2 out]
        n21 = property on="MaxScanMirror" class="DigNum (strict)"("DisabledEnum"=w29) -> ()  [unwired: 2 in, 2 out]
        n22 = property on="@ max Z" class="DigNum (strict)"("DisabledEnum"=w29) -> ()  [unwired: 2 in, 2 out]
        n23 = property on="@ min Z" class="DigNum (strict)"("DisabledEnum"=w29) -> ()  [unwired: 2 in, 2 out]
        n24 = property on="Amplitude" class="DigNum (strict)"("DisabledEnum"=w27) -> ()  [unwired: 2 in, 2 out]
        n25 = property on="MinScanMirror" class="DigNum (strict)"("DisabledEnum"=w29) -> ()  [unwired: 2 in, 2 out]
        n26 = property on="set@maxZ" class="Bool"("DisabledEnum"=w29) -> ()  [unwired: 2 in, 2 out]
        n27 = property on="PiezoStartMicrometres" class="DigNum (strict)"("DisabledEnum"=w29) -> ()  [unwired: 2 in, 2 out]
        n28 = property on="set@minZ" class="Bool"("DisabledEnum"=w29) -> ()  [unwired: 2 in, 2 out]
        n29 = property on="PiezoEndMicrometres" class="DigNum (strict)"("DisabledEnum"=w29) -> ()  [unwired: 2 in, 2 out]
        n30 = property on="Z Mirror Control" class="Enum (strict)"("Value"=enum16{"manual", "automatic"}."manual") -> ()  [unwired: 2 in, 2 out]
        n31 = property on="Offset" class="DigNum (strict)"("DisabledEnum"=w27) -> ()  [unwired: 2 in, 2 out]
        n32 = property on="Phase Shift (µS)" class="Slide (strict)"("DisabledEnum"=w27) -> ()  [unwired: 2 in, 2 out]
        n33 = property on="setPiezoEnd" class="Bool"("DisabledEnum"=w29) -> ()  [unwired: 2 in, 2 out]
        n34 = property on="setPiezoStart" class="Bool"("DisabledEnum"=w29) -> ()  [unwired: 2 in, 2 out]
        n35 = property on="setPosition1" class="Bool"("DisabledEnum"=w29) -> ()  [unwired: 2 in, 2 out]
        n36 = property on="setPosition2" class="Bool"("DisabledEnum"=w29) -> ()  [unwired: 2 in, 2 out]
        n37 = property on="StopSinglePlaneScan" class="Bool"("DisabledEnum"=w27) -> ()  [unwired: 2 in, 2 out]
        n38 = property on="setScanMirrorMax" class="Bool"("DisabledEnum"=w29) -> ()  [unwired: 2 in, 2 out]
        n39 = property on="setScanMirrorMin" class="Bool"("DisabledEnum"=w29) -> ()  [unwired: 2 in, 2 out]
        n40 = property on="Time Interval  Between Repeats (µS)" class="DigNum (strict)"("DisabledEnum"=w27) -> ()  [unwired: 2 in, 2 out]
        n41 = property on="Number of Repetitions" class="DigNum (strict)"("DisabledEnum"=w27) -> ()  [unwired: 2 in, 2 out]
        n42 = property on="StartSinglePlaneScan" class="Bool"("DisabledEnum"=w27) -> ()  [unwired: 2 in, 2 out]
        n43 = property on="Apply ex/det correction" class="Enum (strict)"("DisabledEnum"=w27) -> ()  [unwired: 2 in, 2 out]
        n44 = property on="addMicroscopeSettings" class="Bool"("DisabledEnum"=w29) -> ()  [unwired: 2 in, 2 out]
        n45 = property on="deleteCurrentMicroscopeSettings" class="Bool"("DisabledEnum"=w29) -> ()  [unwired: 2 in, 2 out]
        n46 = property on="applyCurrentMicroscopeSettings" class="Bool"("DisabledEnum"=w29) -> ()  [unwired: 2 in, 2 out]
        n47 = property on="loadMicroscopeSettings" class="Bool"("DisabledEnum"=w29) -> ()  [unwired: 2 in, 2 out]
        n48 = property on="saveMicroscopeSettings" class="Bool"("DisabledEnum"=w29) -> ()  [unwired: 2 in, 2 out]
        n49 = property on="Laser" class="Enum (strict)"("DisabledEnum"=w29) -> ()  [unwired: 2 in, 2 out]
        n50 = property on="StartMultiDScan" class="Bool"("DisabledEnum"=w27) -> ()  [unwired: 2 in, 2 out]
        n51 = property on="Adjusted Scan Mirror Voltage" class="DigNum (strict)"("DisabledEnum"=w29) -> ()  [unwired: 2 in, 2 out]
        n52 = property on="Z Mirror Voltage" class="DigNum (strict)"("DisabledEnum"=w29) -> ()  [unwired: 2 in, 2 out]
        n53 = property on="StopMultiDScan" class="Bool"("DisabledEnum"=w27) -> ()  [unwired: 2 in, 2 out]
        n54 = property on="Z Mirror Control" class="Enum (strict)"("DisabledEnum"=w29) -> ()  [unwired: 2 in, 2 out]
      }
      event "exit": Value Change {
        n55 = event-data() -> ()  [unwired: 1 in, 1 out]
        n56 = shared-variable ".\\SharedVariables.lvlib\\StopSinglePlaneScan"("exit") -> ()  [unwired: 1 in, 1 out]
        n57 = shared-variable ".\\SharedVariables.lvlib\\StopScanMirrorManualControl"("exit") -> ()  [unwired: 1 in, 1 out]
        n58 = shared-variable ".\\SharedVariables.lvlib\\StopMultiDScan"("exit") -> ()  [unwired: 1 in, 1 out]
      }
      event "Mode": Value Change {
        n59 = event-data() -> ()  [unwired: 1 in, 1 out]
        n60 = case shown="\"Single Plane Scan\"" "Mode" {
          tunnel: w41 -> [w49 w60 w66]
          tunnel: w40 -> [w48 w59 w65]
          tunnel: [w47 w58 w64] -> w39
          frame "Manual", Default {
            w43 = T17."Enabled" ("Disabled")
            w46 = T17."Disabled and Grayed Out" ("Disabled")
            n61 = property on="Z Mirror Control" class="Enum (strict)"("Value"=enum16{"manual", "automatic"}."manual" ("Z Mirror Control")) -> ()  [unwired: 2 in, 2 out]
            n62 = property on="Scan Mirror 2" class="DigNum (strict)"("DisabledEnum"=w43) -> ()  [unwired: 2 in, 2 out]
            n63 = property on="Scan Mirror 1" class="DigNum (strict)"("DisabledEnum"=w43) -> ()  [unwired: 2 in, 2 out]
            n64 = property on="Z offset 2" class="DigNum (strict)"("DisabledEnum"=w43) -> ()  [unwired: 2 in, 2 out]
            n65 = property on="Z offset 1" class="DigNum (strict)"("DisabledEnum"=w43) -> ()  [unwired: 2 in, 2 out]
            n66 = property on="Sample Rate (kHz)" class="DigNum (strict)"("DisabledEnum"=w46) -> ()  [unwired: 2 in, 2 out]
            n67 = Enqueue Element(queue=w49, element="manual", error in (no error)=w48) -> (error out=w47:errorcluster)  [unwired: 1 in, 2 out]
            n68 = property on="Piezo Position (µm)" class="Slide (strict)"("DisabledEnum"=w43) -> ()  [unwired: 2 in, 2 out]
            n69 = property on="Mirror Voltage" class="Slide (strict)"("DisabledEnum"=w43) -> ()  [unwired: 2 in, 2 out]
            n70 = property on="Mirror Offset" class="Slide (strict)"("DisabledEnum"=w43) -> ()  [unwired: 2 in, 2 out]
            n71 = property on="Z Mirror Gain" class="Slide (strict)"("DisabledEnum"=w43) -> ()  [unwired: 2 in, 2 out]
            n72 = property on="Lens 2" class="Slide (strict)"("DisabledEnum"=w43) -> ()  [unwired: 2 in, 2 out]
            n73 = property on="Lens 1" class="Slide (strict)"("DisabledEnum"=w43) -> ()  [unwired: 2 in, 2 out]
            n74 = property on="Sweep Time (µS)" class="DigNum (strict)"("DisabledEnum"=w46) -> ()  [unwired: 2 in, 2 out]
            n75 = shared-variable ".\\SharedVariables.lvlib\\StopSinglePlaneScan"(TRUE ("StopSinglePlaneScan")) -> ()  [unwired: 1 in, 1 out]
            n76 = property on="Phase Shift (µS)" class="Slide (strict)"("DisabledEnum"=w46) -> ()  [unwired: 2 in, 2 out]
            n77 = shared-variable ".\\SharedVariables.lvlib\\StopMultiDScan"(TRUE ("StopMultiDScan")) -> ()  [unwired: 1 in, 1 out]
            n78 = property on="Sweep Interval (µS)" class="DigNum (strict)"("DisabledEnum"=w46) -> ()  [unwired: 2 in, 2 out]
            n79 = property on="MaxScanMirror" class="DigNum (strict)"("DisabledEnum"=w43) -> ()  [unwired: 2 in, 2 out]
            n80 = property on="@ max Z" class="DigNum (strict)"("DisabledEnum"=w43) -> ()  [unwired: 2 in, 2 out]
            n81 = property on="@ min Z" class="DigNum (strict)"("DisabledEnum"=w43) -> ()  [unwired: 2 in, 2 out]
            n82 = property on="Amplitude" class="DigNum (strict)"("DisabledEnum"=w46) -> ()  [unwired: 2 in, 2 out]
            n83 = property on="MinScanMirror" class="DigNum (strict)"("DisabledEnum"=w43) -> ()  [unwired: 2 in, 2 out]
            n84 = property on="set@maxZ" class="Bool"("DisabledEnum"=w43) -> ()  [unwired: 2 in, 2 out]
            n85 = property on="PiezoEndMicrometres" class="DigNum (strict)"("DisabledEnum"=w43) -> ()  [unwired: 2 in, 2 out]
            n86 = property on="set@minZ" class="Bool"("DisabledEnum"=w43) -> ()  [unwired: 2 in, 2 out]
            n87 = property on="PiezoStartMicrometres" class="DigNum (strict)"("DisabledEnum"=w43) -> ()  [unwired: 2 in, 2 out]
            n88 = property on="Offset" class="DigNum (strict)"("DisabledEnum"=w46) -> ()  [unwired: 2 in, 2 out]
            n89 = property on="setPiezoEnd" class="Bool"("DisabledEnum"=w43) -> ()  [unwired: 2 in, 2 out]
            n90 = property on="setPiezoStart" class="Bool"("DisabledEnum"=w43) -> ()  [unwired: 2 in, 2 out]
            n91 = property on="setPosition1" class="Bool"("DisabledEnum"=w43) -> ()  [unwired: 2 in, 2 out]
            n92 = property on="setPosition2" class="Bool"("DisabledEnum"=w43) -> ()  [unwired: 2 in, 2 out]
            n93 = property on="StopSinglePlaneScan" class="Bool"("DisabledEnum"=w46) -> ()  [unwired: 2 in, 2 out]
            n94 = property on="setScanMirrorMax" class="Bool"("DisabledEnum"=w43) -> ()  [unwired: 2 in, 2 out]
            n95 = property on="setScanMirrorMin" class="Bool"("DisabledEnum"=w43) -> ()  [unwired: 2 in, 2 out]
            n96 = property on="Apply ex/det correction" class="Enum (strict)"("DisabledEnum"=w46) -> ()  [unwired: 2 in, 2 out]
            n97 = property on="StartSinglePlaneScan" class="Bool"("DisabledEnum"=w46) -> ()  [unwired: 2 in, 2 out]
            n98 = property on="addMicroscopeSettings" class="Bool"("DisabledEnum"=w43) -> ()  [unwired: 2 in, 2 out]
            n99 = property on="deleteCurrentMicroscopeSettings" class="Bool"("DisabledEnum"=w43) -> ()  [unwired: 2 in, 2 out]
            n100 = property on="applyCurrentMicroscopeSettings" class="Bool"("DisabledEnum"=w43) -> ()  [unwired: 2 in, 2 out]
            n101 = property on="loadMicroscopeSettings" class="Bool"("DisabledEnum"=w43) -> ()  [unwired: 2 in, 2 out]
            n102 = property on="saveMicroscopeSettings" class="Bool"("DisabledEnum"=w43) -> ()  [unwired: 2 in, 2 out]
            n103 = property on="Laser" class="Enum (strict)"("DisabledEnum"=w43) -> ()  [unwired: 2 in, 2 out]
            n104 = property on="Adjusted Scan Mirror Voltage" class="DigNum (strict)"("DisabledEnum"=w43) -> ()  [unwired: 2 in, 2 out]
            n105 = property on="Z Mirror Voltage" class="DigNum (strict)"("DisabledEnum"=w43) -> ()  [unwired: 2 in, 2 out]
            n106 = property on="Number of Z Slices" class="DigNum (strict)"("DisabledEnum"=w43) -> ()  [unwired: 2 in, 2 out]
            n107 = property on="Z Mirror Control" class="Enum (strict)"("DisabledEnum"=w43) -> ()  [unwired: 2 in, 2 out]
            n108 = property on="StartMultiDScan" class="Bool"("DisabledEnum"=w46) -> ()  [unwired: 2 in, 2 out]
            n109 = property on="StopMultiDScan" class="Bool"("DisabledEnum"=w46) -> ()  [unwired: 2 in, 2 out]
            n110 = property on="Number of Repetitions" class="DigNum (strict)"("DisabledEnum"=w46) -> ()  [unwired: 2 in, 2 out]
            n111 = property on="Time Interval  Between Stacks (µS)" class="DigNum (strict)"("DisabledEnum"=w46) -> ()  [unwired: 2 in, 2 out]
          }
          frame "Single Plane Scan" {
            w52 = T17."Enabled" ("Disabled")
            n112 = local read "MaxScanMirror"() -> (w55:T3)
            n113 = local read "MinScanMirror"() -> (w54:T3)
            n114 = property on="Phase Shift (µS)" class="Slide (strict)"("DisabledEnum"=w52) -> ()  [unwired: 2 in, 2 out]
            n115 = Subtract(x=w55, y=w54) -> (x-y=w53:T3)
            n116 = property on="Amplitude" class="DigNum (strict)"("DisabledEnum"=w52) -> ()  [unwired: 2 in, 2 out]
            n117 = property on="Sample Rate (kHz)" class="DigNum (strict)"("DisabledEnum"=w52) -> ()  [unwired: 2 in, 2 out]
            n118 = local write "Amplitude"(w53) -> ()
            n119 = local write "Offset"(w54) -> ()
            n120 = Flush Queue(queue=w60, error in (no error)=w59) -> (error out=w58:errorcluster)  [unwired: 2 out]
            n121 = property on="Sweep Interval (µS)" class="DigNum (strict)"("DisabledEnum"=w52) -> ()  [unwired: 2 in, 2 out]
            n122 = property on="Sweep Time (µS)" class="DigNum (strict)"("DisabledEnum"=w52) -> ()  [unwired: 2 in, 2 out]
            n123 = shared-variable ".\\SharedVariables.lvlib\\StopScanMirrorManualControl"(TRUE ("StopScanMirrorManualControl")) -> ()  [unwired: 1 in, 1 out]
            n124 = property on="Offset" class="DigNum (strict)"("DisabledEnum"=w52) -> ()  [unwired: 2 in, 2 out]
            n125 = shared-variable ".\\SharedVariables.lvlib\\StopMultiDScan"(TRUE ("StopMultiDScan")) -> ()  [unwired: 1 in, 1 out]
            n126 = property on="StopSinglePlaneScan" class="Bool"("DisabledEnum"=w52) -> ()  [unwired: 2 in, 2 out]
            n127 = property on="StartSinglePlaneScan" class="Bool"("DisabledEnum"=w52) -> ()  [unwired: 2 in, 2 out]
          }
          frame "Multi-Dimensional Scan" {
            w68 = T17."Enabled" ("Disabled")
            w62 = T17."Disabled and Grayed Out" ("Disabled")
            n128 = property on="Scan Mirror 1" class="DigNum (strict)"("DisabledEnum"=w62) -> ()  [unwired: 2 in, 2 out]
            n129 = property on="Scan Mirror 2" class="DigNum (strict)"("DisabledEnum"=w62) -> ()  [unwired: 2 in, 2 out]
            n130 = property on="Z offset 1" class="DigNum (strict)"("DisabledEnum"=w62) -> ()  [unwired: 2 in, 2 out]
            n131 = property on="Z offset 2" class="DigNum (strict)"("DisabledEnum"=w62) -> ()  [unwired: 2 in, 2 out]
            n132 = Flush Queue(queue=w66, error in (no error)=w65) -> (error out=w64:errorcluster)  [unwired: 2 out]
            n133 = call "DAQ Assistant"("data"=digitalwaveform[] [{"t0"=timestamp(0 s since 1904-01-01), "dt"=0.0, "Y"={"transitions"=[0, 1, 2, 3, 4], "data"=[[0], [0], [0], [0], [0]]}, "error"={"status"=FALSE, "code"=37421928, "source"=""}}, {"t0"=timestamp(0 s since 1904-01-01), "dt"=0.0, "Y"={"transitions"=[0, 1, 2, 3, 4], "data"=[[0], [0], [0], [0], [0]]}, "error"={"status"=FALSE, "code"=37421928, "source"=""}}]) -> ()  [unwired: 17 in, 2 out]
            n134 = property on="Mirror Voltage" class="Slide (strict)"("DisabledEnum"=w62) -> ()  [unwired: 2 in, 2 out]
            n135 = property on="Piezo Position (µm)" class="Slide (strict)"("DisabledEnum"=w62) -> ()  [unwired: 2 in, 2 out]
            n136 = property on="Mirror Offset" class="Slide (strict)"("DisabledEnum"=w62) -> ()  [unwired: 2 in, 2 out]
            n137 = property on="Z Mirror Gain" class="Slide (strict)"("DisabledEnum"=w62) -> ()  [unwired: 2 in, 2 out]
            n138 = property on="Lens 1" class="Slide (strict)"("DisabledEnum"=w62) -> ()  [unwired: 2 in, 2 out]
            n139 = property on="Lens 2" class="Slide (strict)"("DisabledEnum"=w62) -> ()  [unwired: 2 in, 2 out]
            n140 = shared-variable ".\\SharedVariables.lvlib\\StopScanMirrorManualControl"(TRUE ("StopScanMirrorManualControl")) -> ()  [unwired: 1 in, 1 out]
            n141 = property on="Sample Rate (kHz)" class="DigNum (strict)"("DisabledEnum"=w62) -> ()  [unwired: 2 in, 2 out]
            n142 = property on="Phase Shift (µS)" class="Slide (strict)"("DisabledEnum"=w62) -> ()  [unwired: 2 in, 2 out]
            n143 = property on="MaxScanMirror" class="DigNum (strict)"("DisabledEnum"=w62) -> ()  [unwired: 2 in, 2 out]
            n144 = property on="@ min Z" class="DigNum (strict)"("DisabledEnum"=w62) -> ()  [unwired: 2 in, 2 out]
            n145 = property on="MinScanMirror" class="DigNum (strict)"("DisabledEnum"=w62) -> ()  [unwired: 2 in, 2 out]
            n146 = property on="@ max Z" class="DigNum (strict)"("DisabledEnum"=w62) -> ()  [unwired: 2 in, 2 out]
            n147 = property on="PiezoStartMicrometres" class="DigNum (strict)"("DisabledEnum"=w62) -> ()  [unwired: 2 in, 2 out]
            n148 = property on="PiezoEndMicrometres" class="DigNum (strict)"("DisabledEnum"=w62) -> ()  [unwired: 2 in, 2 out]
            n149 = property on="set@maxZ" class="Bool"("DisabledEnum"=w62) -> ()  [unwired: 2 in, 2 out]
            n150 = property on="set@minZ" class="Bool"("DisabledEnum"=w62) -> ()  [unwired: 2 in, 2 out]
            n151 = shared-variable ".\\SharedVariables.lvlib\\StopSinglePlaneScan"(TRUE ("StopSinglePlaneScan")) -> ()  [unwired: 1 in, 1 out]
            n152 = property on="Sweep Interval (µS)" class="DigNum (strict)"("DisabledEnum"=w62) -> ()  [unwired: 2 in, 2 out]
            n153 = property on="Sweep Time (µS)" class="DigNum (strict)"("DisabledEnum"=w62) -> ()  [unwired: 2 in, 2 out]
            n154 = property on="setPiezoEnd" class="Bool"("DisabledEnum"=w62) -> ()  [unwired: 2 in, 2 out]
            n155 = property on="setPiezoStart" class="Bool"("DisabledEnum"=w62) -> ()  [unwired: 2 in, 2 out]
            n156 = property on="setPosition1" class="Bool"("DisabledEnum"=w62) -> ()  [unwired: 2 in, 2 out]
            n157 = property on="setPosition2" class="Bool"("DisabledEnum"=w62) -> ()  [unwired: 2 in, 2 out]
            n158 = property on="setScanMirrorMax" class="Bool"("DisabledEnum"=w62) -> ()  [unwired: 2 in, 2 out]
            n159 = property on="setScanMirrorMin" class="Bool"("DisabledEnum"=w62) -> ()  [unwired: 2 in, 2 out]
            n160 = property on="Offset" class="DigNum (strict)"("DisabledEnum"=w62) -> ()  [unwired: 2 in, 2 out]
            n161 = property on="Amplitude" class="DigNum (strict)"("DisabledEnum"=w62) -> ()  [unwired: 2 in, 2 out]
            n162 = property on="addMicroscopeSettings" class="Bool"("DisabledEnum"=w62) -> ()  [unwired: 2 in, 2 out]
            n163 = property on="applyCurrentMicroscopeSettings" class="Bool"("DisabledEnum"=w62) -> ()  [unwired: 2 in, 2 out]
            n164 = property on="Z Mirror Control" class="Enum (strict)"("DisabledEnum"=w62) -> ()  [unwired: 2 in, 2 out]
            n165 = property on="Laser" class="Enum (strict)"("DisabledEnum"=w62) -> ()  [unwired: 2 in, 2 out]
            n166 = property on="Apply ex/det correction" class="Enum (strict)"("DisabledEnum"=w62) -> ()  [unwired: 2 in, 2 out]
            n167 = property on="Adjusted Scan Mirror Voltage" class="DigNum (strict)"("DisabledEnum"=w62) -> ()  [unwired: 2 in, 2 out]
            n168 = property on="Number of Z Slices" class="DigNum (strict)"("DisabledEnum"=w62) -> ()  [unwired: 2 in, 2 out]
            n169 = property on="Mirror Voltage" class="Slide (strict)"("DisabledEnum"=w62) -> ()  [unwired: 2 in, 2 out]
            n170 = property on="StartSinglePlaneScan" class="Bool"("DisabledEnum"=w62) -> ()  [unwired: 2 in, 2 out]
            n171 = property on="StopSinglePlaneScan" class="Bool"("DisabledEnum"=w62) -> ()  [unwired: 2 in, 2 out]
            n172 = property on="deleteCurrentMicroscopeSettings" class="Bool"("DisabledEnum"=w68) -> ()  [unwired: 2 in, 2 out]
            n173 = property on="loadMicroscopeSettings" class="Bool"("DisabledEnum"=w68) -> ()  [unwired: 2 in, 2 out]
            n174 = property on="saveMicroscopeSettings" class="Bool"("DisabledEnum"=w68) -> ()  [unwired: 2 in, 2 out]
            n175 = property on="StartMultiDScan" class="Bool"("DisabledEnum"=w68) -> ()  [unwired: 2 in, 2 out]
            n176 = property on="StopMultiDScan" class="Bool"("DisabledEnum"=w68) -> ()  [unwired: 2 in, 2 out]
            n177 = property on="Number of Repetitions" class="DigNum (strict)"("DisabledEnum"=w68) -> ()  [unwired: 2 in, 2 out]
            n178 = property on="Time Interval  Between Stacks (µS)" class="DigNum (strict)"("DisabledEnum"=w68) -> ()  [unwired: 2 in, 2 out]
          }
        }
      }
      event "StartSinglePlaneScan": Value Change {
        # "Generate the data here."
        n179 = event-data() -> ()  [unwired: 1 in, 1 out]
        n180 = Enqueue Element(queue=w75, element="SinglePlaneScan", error in (no error)=w74) -> (error out=w73:errorcluster)  [unwired: 1 in, 2 out]
        n181 = property on="StopSinglePlaneScan" class="Bool"("DisabledEnum"=T17."Enabled" ("Disabled")) -> ()  [unwired: 2 in, 2 out]
        n182 = property on="StartSinglePlaneScan" class="Bool"("DisabledEnum"=T17."Disabled and Grayed Out" ("Disabled")) -> ()  [unwired: 2 in, 2 out]
      }
      event "StopSinglePlaneScan": Value Change {
        n183 = event-data() -> ()  [unwired: 1 in, 1 out]
        n184 = shared-variable ".\\SharedVariables.lvlib\\StopSinglePlaneScan"("StopSinglePlaneScan") -> ()  [unwired: 1 in, 1 out]
        n185 = Flush Queue(queue=w81, error in (no error)=w80) -> (error out=w79:errorcluster)  [unwired: 2 out]
        n186 = property on="StartSinglePlaneScan" class="Bool"("DisabledEnum"=T17."Enabled" ("Disabled")) -> ()  [unwired: 2 in, 2 out]
        n187 = property on="StopSinglePlaneScan" class="Bool"("DisabledEnum"=T17."Disabled and Grayed Out" ("Disabled")) -> ()  [unwired: 2 in, 2 out]
      }
      event "StartMultiDScan": Value Change {
        n188 = event-data() -> ()  [unwired: 1 in, 1 out]
        n189 = Enqueue Element(queue=w89, element="MultiDScan", error in (no error)=w88) -> (error out=w87:errorcluster)  [unwired: 1 in, 2 out]
        n190 = property on="StopMultiDScan" class="Bool"("DisabledEnum"=T17."Enabled" ("Disabled")) -> ()  [unwired: 2 in, 2 out]
        n191 = property on="StartMultiDScan" class="Bool"("DisabledEnum"=T17."Disabled and Grayed Out" ("Disabled")) -> ()  [unwired: 2 in, 2 out]
      }
      event "StopMultiDScan": Value Change {
        n192 = event-data() -> ()  [unwired: 1 in, 1 out]
        n193 = Flush Queue(queue=w96, error in (no error)=w95) -> (error out=w94:errorcluster)  [unwired: 2 out]
        n194 = property on="StartMultiDScan" class="Bool"("DisabledEnum"=T17."Enabled" ("Disabled")) -> ()  [unwired: 2 in, 2 out]
        n195 = property on="StopMultiDScan" class="Bool"("DisabledEnum"=T17."Disabled and Grayed Out" ("Disabled")) -> ()  [unwired: 2 in, 2 out]
        n196 = shared-variable ".\\SharedVariables.lvlib\\StopMultiDScan"(TRUE ("StopMultiDScan")) -> ()  [unwired: 1 in, 1 out]
      }
      event "Z Mirror Control": Value Change {
        n197 = event-data() -> ()  [unwired: 1 in, 1 out]
        n198 = case shown="\"manual\", Default" w97 {
          frame "manual", Default {
            w99 = T17."Disabled and Grayed Out" ("Disabled")
            n199 = property on="Mirror Offset" class="Slide (strict)"("DisabledEnum"=w99) -> ()  [unwired: 2 in, 2 out]
            n200 = property on="Z Mirror Gain" class="Slide (strict)"("DisabledEnum"=w99) -> ()  [unwired: 2 in, 2 out]
            n201 = property on="setPosition1" class="Bool"("DisabledEnum"=w99) -> ()  [unwired: 2 in, 2 out]
            n202 = property on="setPosition2" class="Bool"("DisabledEnum"=w99) -> ()  [unwired: 2 in, 2 out]
            n203 = property on="Apply ex/det correction" class="Enum (strict)"("DisabledEnum"=T17."Enabled" ("Disabled")) -> ()  [unwired: 2 in, 2 out]
          }
          frame "automatic" {
            w101 = T17."Enabled" ("Disabled")
            n204 = property on="Z Mirror Gain" class="Slide (strict)"("DisabledEnum"=w101) -> ()  [unwired: 2 in, 2 out]
            n205 = property on="Mirror Offset" class="Slide (strict)"("DisabledEnum"=w101) -> ()  [unwired: 2 in, 2 out]
            n206 = property on="setPosition1" class="Bool"("DisabledEnum"=w101) -> ()  [unwired: 2 in, 2 out]
            n207 = property on="setPosition2" class="Bool"("DisabledEnum"=w101) -> ()  [unwired: 2 in, 2 out]
            n208 = property on="Apply ex/det correction" class="Enum (strict)"("DisabledEnum"=T17."Disabled and Grayed Out" ("Disabled")) -> ()  [unwired: 2 in, 2 out]
          }
        }
      }
      event "Mirror Voltage", "Mirror Offset": Value Change {
        n209 = event-data() -> ()  [unwired: 1 in, 1 out]
        n210 = shared-variable ".\\SharedVariables.lvlib\\Laser"("Laser") -> ()  [unwired: 1 in, 1 out]
        n211 = call "mirrorCorrections.vi"("Scan Mirror Min"="MinScanMirror", "Beam@maxZ"="@ max Z", "Z Mirror Offset"="Mirror Offset", "Z Mirror Gain"="Z Mirror Gain", "Piezo Position (µm)"="Piezo Position (µm)", "Piezo Min (µm)"="PiezoStartMicrometres", "Piezo Max (µm)"="PiezoEndMicrometres", "Scan Mirror Max"="MaxScanMirror", "Scan Mirror Voltage"="Mirror Voltage", "Scan Mirror Position 2"="Scan Mirror 2", "Z Mirror Control"=w115, "Z Offset Position 2"="Z offset 2", "Apply ex/det correction"=w114) -> ("Adjusted Scan Mirror Voltage"=w113:T3, "Z Mirror Voltage"=w112:T3)  [unwired: 13 in]
        "Adjusted Scan Mirror Voltage" <- w113
        "Z Mirror Voltage" <- w112
        n212 = shared-variable ".\\SharedVariables.lvlib\\ScanMirrorVoltage"(w113) -> ()  [unwired: 1 in, 1 out]
        n213 = shared-variable ".\\SharedVariables.lvlib\\ZMirrorVoltage"(w112) -> ()  [unwired: 1 in, 1 out]
        n214 = shared-variable ".\\SharedVariables.lvlib\\PiezoMicrometres"("Piezo Position (µm)") -> ()  [unwired: 1 in, 1 out]
        n215 = In Range and Coerce(upper limit=T5 3.0, x="Lens 1", lower limit=T5 0.0) -> (coerced(x)=w109:T5)  [unwired: 1 out]
        n216 = In Range and Coerce(upper limit=T5 3.0, x="Lens 2", lower limit=T5 0.0) -> (coerced(x)=w110:T5)  [unwired: 1 out]
        n217 = shared-variable ".\\SharedVariables.lvlib\\Lens1"(w109) -> ()  [unwired: 1 in, 1 out]
        n218 = shared-variable ".\\SharedVariables.lvlib\\Lens2"(w110) -> ()  [unwired: 1 in, 1 out]
      }
      event "setScanMirrorMax": Value Change {
        n219 = event-data() -> ()  [unwired: 1 in, 1 out]
        n220 = local read "Mirror Voltage"() -> (w128:dbl)
        n221 = local write "MaxScanMirror"(w128) -> ()
      }
      event "setScanMirrorMin": Value Change {
        n222 = event-data() -> ()  [unwired: 1 in, 1 out]
        n223 = local read "Mirror Voltage"() -> (w130:dbl)
        n224 = local write "MinScanMirror"(w130) -> ()
      }
      event "setPosition1": Value Change {
        n225 = event-data() -> ()  [unwired: 1 in, 1 out]
        n226 = local read "Mirror Voltage"() -> (w133:dbl)
        n227 = local read "Mirror Offset"() -> (w132:dbl)
        n228 = local write "Z offset 1"(w132) -> ()
        n229 = local write "Scan Mirror 1"(w133) -> ()
      }
      event "setPosition2": Value Change {
        n230 = event-data() -> ()  [unwired: 1 in, 1 out]
        n231 = local read "Mirror Voltage"() -> (w136:dbl)
        n232 = local read "Mirror Offset"() -> (w135:dbl)
        n233 = local write "Scan Mirror 2"(w136) -> ()
        n234 = local write "Z offset 2"(w135) -> ()
      }
      event "setPiezoStart": Value Change {
        n235 = event-data() -> ()  [unwired: 1 in, 1 out]
        n236 = local read "Piezo Position (µm)"() -> (w138:T8)
        n237 = local write "PiezoStartMicrometres"(w138) -> ()
      }
      event "setPiezoEnd": Value Change {
        n238 = event-data() -> ()  [unwired: 1 in, 1 out]
        n239 = local read "Piezo Position (µm)"() -> (w140:T8)
        n240 = local write "PiezoEndMicrometres"(w140) -> ()
      }
      event "set@maxZ": Value Change {
        n241 = event-data() -> ()  [unwired: 1 in, 1 out]
        n242 = local read "Mirror Voltage"() -> (w142:dbl)
        n243 = local write "@ max Z"(w142) -> ()
      }
      event "set@minZ": Value Change {
        n244 = event-data() -> ()  [unwired: 1 in, 1 out]
        n245 = local read "Mirror Voltage"() -> (w144:dbl)
        n246 = local write "@ min Z"(w144) -> ()
      }
      event "addMicroscopeSettings": Value Change {
        n247 = event-data() -> ()  [unwired: 1 in, 1 out]
        n248 = local read "MaxScanMirror"() -> (w165:T3)
        n249 = local read "MinScanMirror"() -> (w164:T3)
        n250 = local read "PiezoStartMicrometres"() -> (w153:T4)
        n251 = local read "PiezoEndMicrometres"() -> (w152:T4)
        n252 = local read "Sweep Interval (µS)"() -> (w168:T2)
        n253 = local read "Number of Z Slices"() -> (w151:i16)
        n254 = local read "Sample Rate (kHz)"() -> (w167:i32)
        n255 = local read "Sweep Time (µS)"() -> (w145:T2)
        n256 = local read "Sweep Time (µS)"() -> (w169:T2)
        n257 = local read "Phase Shift (µS)"() -> (w166:i32)
        n258 = local read "Mirror Offset"() -> (w146:dbl)
        n259 = local read "Z Mirror Gain"() -> (w162:T6)
        n260 = local read "Scan Mirror 1"() -> (w161:T3)
        n261 = local read "Scan Mirror 2"() -> (w159:T3)
        n262 = local read "Z offset 1"() -> (w160:T9)
        n263 = local read "Z offset 2"() -> (w158:T9)
        n264 = local read "@ min Z"() -> (w155:T3)
        n265 = local read "@ max Z"() -> (w154:T3)
        n266 = Subtract(x=w165, y=w164) -> (x-y=w163:T3)
        n267 = local read "Lens 1"() -> (w157:T5)
        n268 = local read "Lens 2"() -> (w156:T5)
        n269 = local read "Laser"() -> (w170:T7)
        n270 = Bundle("Laser"=w170, "Sweep Time (µS)"=w169, "Sweep Interval (µS)"=w168, "Sample Rate (kHz)"=w167, "Phase Shift (µS)"=w166, "MaxScanMirror"=w165, "MinScanMirror"=w164, "MaxScanMirror"=w163, "Mirror Offset"=w146, "Z Mirror Gain"=w162, "Scan Mirror 1"=w161, "Z offset 1"=w160, "Scan Mirror 2"=w159, "Z offset 2"=w158, "Lens 1"=w157, "Lens 2"=w156, "@ min Z"=w155, "@ max Z"=w154, "PiezoStartMicrometres"=w153, "PiezoEndMicrometres"=w152, "Number of Z Slices"=w151, "Sweep Time (µS)"=w145, "Apply ex/det correction"=w150) -> ()  [unwired: 1 in, 1 out]
        n271 = Index Array(array=w171, index=0) -> (element=w147:T10)
        n272 = call "Waveform_Generation2.vi"() -> ("output cluster"=w149:T14)  [unwired: 10 in]
        n273 = Bundle By Name(cluster=w147, "Laser"=w170, "Sweep Time (µS)"=w169, "Sweep Interval (µS)"=w168, "Sample Rate (kHz)"=w167, "Camera Phase Shift (µS)"=w166, "Scan Mirror Max"=w165, "Scan Mirror Min"=w164, "Scan Mirror Amplitude"=w163, "Z Offset"=w146, "Z Gain"=w162, "Scan Mirror Position 1"=w161, "Z Offset Position 1"=w160, "Scan Mirror Position 2"=w159, "Z Offset Position 2"=w158, "Tuneable Lens 1"=w157, "Tuneable Lens 2"=w156, "Beam @ min Z"=w155, "Beam @ max Z"=w154, "Piezo Start (µm)"=w153, "Piezo End (µm)"=w152, "Number Z Slices"=w151, "Filter Wheel Position"=w145, "Apply ex/det correction"=w150, "waveforms"=w149) -> (w148:T10)
        n274 = Build Array (concatenate)(w171, w148) -> (w172:T10[])
        n275 = Array Size(array=w172) -> (size(s)=w175:i32)
        n276 = Decrement(x=w175) -> (x-1=w176:i32)
        n277 = Build Array(w176) -> (w174:i32[])
        n278 = property on="Microscope Settings" class="Arr (strict)"("Index Values"=w174) -> ()  [unwired: 2 in, 2 out]
      }
      event "deleteCurrentMicroscopeSettings": Value Change {
        n279 = event-data() -> ()  [unwired: 1 in, 1 out]
        n280 = Two Button Dialog(message="Delete current setting from array", 1:"No" ("F button name (\"Cancel\")"), 2:"Yes" ("T button name (\"OK\")")) -> (T button?=w179:bool)
        n281 = case shown="True" w179 {
          tunnel: w177 -> [w183 w188]
          tunnel: [w183 w184] -> w178
          frame False {
          }
          frame True {
            n282 = property on="Microscope Settings" class="Arr (strict)"() -> ("Index Values"=w187:u32[])  [unwired: 2 in, 2 out]
            n283 = for {
              tunnel: w187 -> [w191] mode=indexing
              tunnel: [w191] -> w186
            }
            n284 = Decrement(x=w186) -> (x-1=w189:u32)
            n285 = Build Array(w189) -> (w185:u32[])
            n286 = Delete From Array(array=w188, length=1) -> (array with subset deleted=w184:T10[])  [unwired: 1 in, 1 out]
            n287 = property on="Microscope Settings" class="Arr (strict)"("Index Values"=w185) -> ()  [unwired: 2 in, 2 out]
          }
        }
      }
      event "applyCurrentMicroscopeSettings": Value Change {
        # "Apply Current Settings"
        n288 = event-data() -> ()  [unwired: 1 in, 1 out]
        n289 = property on="Microscope Settings" class="Arr (strict)"() -> ("Index Values"=w215:u32[])  [unwired: 2 in, 2 out]
        n290 = for {
          tunnel: w215 -> [w217] mode=indexing
          tunnel: [w217] -> w216
        }
        n291 = Index Array(array=w213, index=w216) -> (element=w214:T10)
        n292 = Unbundle By Name(w214) -> ("Laser"=w212:T7, "Sweep Time (µS)"=w211:T2, "Sweep Interval (µS)"=w210:T2, "Sample Rate (kHz)"=w209:dbl, "Camera Phase Shift (µS)"=w208:T11, "Scan Mirror Max"=w207:T3, "Scan Mirror Min"=w206:T3, "Z Offset"=w193:T9, "Z Gain"=w192:T12, "Scan Mirror Position 1"=w205:T3, "Z Offset Position 1"=w204:T9, "Scan Mirror Position 2"=w203:T3, "Z Offset Position 2"=w202:T9, "Tuneable Lens 1"=w201:T13, "Tuneable Lens 2"=w200:T13, "Beam @ min Z"=w198:T3, "Beam @ max Z"=w199:T3, "Piezo Start (µm)"=w196:T4, "Piezo End (µm)"=w197:T4, "Number Z Slices"=w195:i16, "Apply ex/det correction"=w194:u16)  [unwired: 2 out]
        n293 = local write "MaxScanMirror"(w207) -> ()
        n294 = local write "Apply ex/det correction"(w194) -> ()
        n295 = local write "PiezoEndMicrometres"(w197) -> ()
        n296 = local write "Number of Z Slices"(w195) -> ()
        n297 = local write "Lens 2"(w200) -> ()
        n298 = local write "@ max Z"(w199) -> ()
        n299 = local write "Lens 1"(w201) -> ()
        n300 = local write "Scan Mirror 1"(w205) -> ()
        n301 = local write "Scan Mirror 2"(w203) -> ()
        n302 = local write "Sample Rate (kHz)"(w209) -> ()
        n303 = local write "Laser"(w212) -> ()
        n304 = local write "Mirror Offset"(w193) -> ()
        n305 = local write "Z Mirror Gain"(w192) -> ()
        n306 = local write "Sweep Time (µS)"(w211) -> ()
        n307 = local write "@ min Z"(w198) -> ()
        n308 = local write "PiezoStartMicrometres"(w196) -> ()
        n309 = local write "MinScanMirror"(w206) -> ()
        n310 = local write "Z offset 2"(w202) -> ()
        n311 = local write "Z offset 1"(w204) -> ()
        n312 = local write "Sweep Interval (µS)"(w210) -> ()
        n313 = local write "Phase Shift (µS)"(w208) -> ()
      }
      event "loadMicroscopeSettings": Value Change {
        n314 = event-data() -> ()  [unwired: 1 in, 1 out]
        n315 = File Dialog(7:"Select Settings File " ("prompt")) -> (0:w223:errorcluster, 3:w221:path)  [unwired: 2 in, 6 out]
        n316 = Index Array(array=w219, index=0) -> (element=w220:T10)
        n317 = case shown="No Error" w223 {
          tunnel: w221 -> [w232 _]
          tunnel: w220 -> [w229 _]
          tunnel: [w225 w240] -> w218
          tunnel: w219 -> [_ w240]
          frame No Error {
            n318 = Open/Create/Replace Datalog(5:w229, 9:enum16{"read/write", "read-only", "write-only"}."read-only" ("access (0:read/write)"), 11:w232) -> (0:w239:errorcluster, 3:w230:refnum<k1>)  [unwired: 2 in, 2 out]
            n319 = Deny Access(4:w239, 6:T18."deny write-only" ("deny mode (0:deny read/write)"), 7:w230) -> (0:w238:errorcluster, 3:w237:refnum<k1>)
            n320 = Get Number of Records(4:w238, 7:w237) -> (0:w228:errorcluster, 2:w235:i64, 3:w236:refnum<k1>)
            n321 = Read Datalog(4:w228, 6:w235, 7:w236) -> (0:w227:errorcluster, 2:w225:T10[], 3:w234:refnum<k1>)
            n322 = Close File(refnum=w234, error in=w227) -> (error out=w233:errorcluster)  [unwired: 1 out]
            n323 = call <vilib>:"General Error Handler.vi"("error in (no error)"=w233) -> ()  [unwired: 5 in, 10 out]
          }
          frame Error {
          }
        }
      }
      event "saveMicroscopeSettings": Value Change {
        n324 = event-data() -> ()  [unwired: 1 in, 1 out]
        n325 = File Dialog(7:"Choose file name and location" ("prompt"), 9:"tunable lens settings.dat" ("default name")) -> (0:w245:errorcluster, 3:w244:path)  [unwired: 1 in, 6 out]
        n326 = Index Array(array=w241, index=0) -> (element=w242:T10)
        n327 = case shown="No Error" w245 {
          tunnel: w244 -> [w250 _]
          tunnel: w242 -> [w249 _]
          tunnel: w241 -> [w248 _]
          frame No Error {
            n328 = Open/Create/Replace Datalog(5:w249, 10:T19."replace or create" ("operation (0:open)"), 11:w250) -> (3:w253:refnum<k1>)  [unwired: 1 in, 4 out]
            n329 = for {
              tunnel: w248 -> [w259] mode=indexing
              tunnel: w253 -> [w258]
              tunnel: [w257] -> w252
              tunnel: [w256] -> w251
              n330 = Write Datalog(6:w259, 7:w258) -> (0:w256:errorcluster, 3:w257:refnum<k1>)  [unwired: 1 in]
            }
            n331 = Close File(refnum=w252, error in=w251) -> (error out=w255:errorcluster)  [unwired: 1 out]
            n332 = call <vilib>:"General Error Handler.vi"("error in (no error)"=w255) -> ()  [unwired: 2 in, 13 out]
          }
          frame Error {
          }
        }
      }
    }
    n333 = shared-variable "My Computer\\SharedVariables.lvlib\\COMport"("COM port") -> ()  [unwired: 1 in, 1 out]
    n334 = Unbundle By Name(w21) -> ("status"=w20:bool)
    n335 = local write "Microscope Settings"(w14) -> ()
    n336 = Or(x=w20, y=w23) -> (x .or. y?=w22:bool)
  }
  n337 = Bundle(ArduinoII."Timed XP", "Master"=T16 {"Current"={"curr_1_value"=0.0, "curr_2_value"=0.0, "curr_3_value"=0.0, "curr_4_value"=0.0, "Write All"=FALSE}, "Boolean Set"={"XY Up"=FALSE, "XY Down"=FALSE, "XY Left"=FALSE, "XY Right"=FALSE, "Z Up"=FALSE, "Z Down"=FALSE}, "Cluster"={"XY Up"=0.0, "XY Down"=0.0, "XY Left"=0.0, "XY Right"=0.0, "Z Up"=0.0, "Z Down"=0.0}, "Timing"={"t1"=0.0, "t2"=0.0, "Timed Experiment"=FALSE}, "Power"={"Power ON"=FALSE, "Power OFF"=FALSE}}) -> (w3:cluster{T15, "Master":T16})  [unwired: 1 in]
  n338 = Obtain Queue(name (unnamed)="PowerDuino", element data type=w3, create if not found? (T)=FALSE) -> (queue out=w2:refnum<queue>, error out=→"error out":errorcluster)  [unwired: 2 in, 1 out]
  n339 = while {
    tunnel: w8 -> [w264]
    tunnel: w2 -> [w260]
    stop <- w261 stop-if-true
    # "This loop is a consumer loop."
    n340 = Dequeue Element(queue=w264) -> (element=w262:string, error out=w263:errorcluster)  [unwired: 2 in, 2 out]
    n341 = case shown="No Error" w263 {
      tunnel: w262 -> [w266 _]
      tunnel: [_ TRUE] -> w261
      tunnel: w260 -> [w265 _]
      frame No Error {
        n342 = case shown="\"MultiDScan\"" w266 {
          tunnel: w265 -> [_ w281 _ _]
          frame "SinglePlaneScan" {
            # "Process the data here."
            n343 = flat-sequence {
              frame #0 {
                n344 = shared-variable ".\\SharedVariables.lvlib\\StopSinglePlaneScan"(FALSE ("StopScan")) -> ()  [unwired: 1 in, 1 out]
              }
              frame #1 {
                n345 = while {
                  stop <- w268 stop-if-true
                  n346 = local read "Z offset 2"() -> (w273:T9)
                  n347 = local read "Mirror Offset"() -> (w272:dbl)
                  n348 = local read "Z Mirror Gain"() -> (w271:T6)
                  n349 = shared-variable ".\\SharedVariables.lvlib\\StopSinglePlaneScan"() -> (w268:bool)  [unwired: 1 in, 1 out]
                  n350 = local read "Piezo Position (µm)"() -> (w270:T8)
                  n351 = local read "@ max Z"() -> (w269:T3)
                  n352 = local read "Laser"() -> (w280:T7)
                  n353 = call "simple_scan_mathscript.vi"("Piezo"=w270, "Beam at max"=w269, "Laser"=w280, "Sweep Interval"="Sweep Interval (µS)", "Z mirror Gain"=w271, "Sample Rate"="Sample Rate (kHz)", "Z mirror offset"=w272, "Sweep Time"="Sweep Time (µS)", "Z offset 2"=w273, "Offset"="Offset", "Amplitude"="Amplitude", "Phase Shift"="Phase Shift (µS)") -> ()
                }
              }
            }
          }
          frame "MultiDScan" {
            n354 = flat-sequence {
              tunnel: [w283] -> w282
              tunnel: w281 -> [w283]
              tunnel: w282 -> [w286]
              frame #0 {
                n355 = shared-variable ".\\SharedVariables.lvlib\\StopMultiDScan"(FALSE ("StopMultiDScan")) -> ()  [unwired: 1 in, 1 out]
              }
              frame #1 {
                n356 = for {
                  N: "Experiment Runs" -> [_]
                  tunnel: "Time Interval  Between Repeats (µS)" -> [w294]
                  tunnel: "Number of Repetitions" -> [w293]
                  tunnel: "Microscope Settings" -> [w292]
                  tunnel: w286 -> [w291]
                  n357 = case shown="True" "Experiment?" {
                    tunnel: w291 -> [_ w299]
                    frame False {
                    }
                    frame True {
                      n358 = Bundle By Name(cluster=T16 {"Current"={"curr_1_value"=0.0, "curr_2_value"=0.0, "curr_3_value"=0.0, "curr_4_value"=0.0, "Write All"=FALSE}, "Boolean Set"={"XY Up"=FALSE, "XY Down"=FALSE, "XY Left"=FALSE, "XY Right"=FALSE, "Z Up"=FALSE, "Z Down"=FALSE}, "Cluster"={"XY Up"=0.0, "XY Down"=0.0, "XY Left"=0.0, "XY Right"=0.0, "Z Up"=0.0, "Z Down"=0.0}, "Timing"={"t1"=30.0, "t2"=60.0, "Timed Experiment"=FALSE}, "Power"={"Power ON"=FALSE, "Power OFF"=FALSE}} ("Master"), "Timing.t1"="t1", "Timing.t2"="t2") -> (w295:T16)
                      n359 = Bundle(ArduinoII."Timed XP", "Master"=w295) -> (w301:cluster{T15, "Master":T16})  [unwired: 1 in]
                      n360 = Enqueue Element(queue=w299, element=w301) -> ()  [unwired: 2 in, 3 out]
                    }
                  }
                  n361 = call "multiD.vi"("Time Interval Between Repeats mS)"=w294, "Number of repetitions"=w293, "Array"=w292) -> ()  [unwired: 9 in]
                }
              }
              frame #2 {
                n362 = property on="StopMultiDScan" class="Bool"("DisabledEnum"=T17."Disabled and Grayed Out" ("Disabled")) -> ()  [unwired: 2 in, 2 out]
                n363 = property on="StartMultiDScan" class="Bool"("DisabledEnum"=T17."Enabled" ("Disabled")) -> ()  [unwired: 2 in, 2 out]
              }
            }
          }
          frame "manual" {
            n364 = call "mirrors_and_piezo_manual_scan.vi"("Stop Button"=FALSE) -> ()  [unwired: 1 in]
          }
          frame "other", Default {
          }
        }
      }
      frame Error {
        # "Return true in any case that should stop the loop."
      }
    }
  }
  n365 = Release Queue(queue=w8, error in (no error)=w11) -> ()  [unwired: 1 in, 3 out]
